vi "Oxford-1820-Main.vi"() -> ()   [LabVIEW 2016]
uses:
  <instrlib>/Mercury iXX/Public/Controls/Unit String.ctl
  <instrlib>/Mercury iXX/Public/Libraries/Heater/Controls/Heater Device (Read).ctl
  <instrlib>/Mercury iXX/Public/Controls/Manufacturing Data.ctl
  <instrlib>/Mercury iXX/Public/Libraries/Heater/Controls/Heater Signals Cluster.ctl
  <instrlib>/Mercury iXX/Public/Libraries/Level Meter/Controls/Level Meter (Read).ctl
  <instrlib>/Mercury iXX/Public/Libraries/Level Meter/Controls/Nitrogen Configuration.ctl
  <instrlib>/Mercury iXX/Public/Libraries/Level Meter/Controls/Frequency Configuration.ctl
  <instrlib>/Mercury iXX/Public/Libraries/Level Meter/Controls/Signals.ctl
  <instrlib>/Mercury iXX/Public/Libraries/Level Meter/Controls/Helium Configuration.ctl
  <instrlib>/Mercury iXX/Public/Libraries/Level Meter/Controls/Resistance Configuration.ctl
  <instrlib>/Mercury iXX/Public/Libraries/Level Meter/Controls/Pre-Pulse.ctl
  <instrlib>/Mercury iXX/Public/Libraries/Level Meter/Controls/Pulse.ctl
  <instrlib>/Mercury iXX/Public/Libraries/Auxiliary/Controls/AUX Device (Read).ctl
  <instrlib>/Mercury iXX/Public/Libraries/Auxiliary/Controls/AUX Signals (Read).ctl
  <instrlib>/Mercury iXX/Public/Libraries/Magnet/Controls/Device (Read).ctl
  <instrlib>/Mercury iXX/Public/Libraries/Magnet/Controls/Signals (Read).ctl
  <instrlib>/Mercury iXX/Public/Libraries/Magnet/Controls/Identifier.ctl
  <instrlib>/Mercury iXX/Public/Libraries/Temperature/Controls/Calibration Cluster.ctl
  <instrlib>/Mercury iXX/Public/Libraries/Temperature/Controls/Calibration Interpolation.ctl
  <instrlib>/Mercury iXX/Public/Libraries/Temperature/Controls/Excitation Cluster.ctl
  <instrlib>/Mercury iXX/Public/Libraries/Temperature/Controls/Excitation Type.ctl
  <instrlib>/Mercury iXX/Public/Libraries/Pressure/Controls/Pressure Signals Cluster.ctl
  <instrlib>/Mercury iXX/Public/Controls/Mercury Reference.ctl
  <instrlib>/Mercury iXX/Public/Controls/Comms Transport Layer.ctl
  <instrlib>/Mercury iXX/Private/Controls/Query Dynamic Reference.ctl
  <userlib>/LevyLab/Oxford 1820 API/Typedefs/Status.ctl
  <instrlib>/Mercury iXX/Public/Libraries/Magnet/Controls/PSU Actions.ctl
  <instrlib>/Mercury iXX/Public/Libraries/System/Controls/User Mode.ctl
  <instrlib>/Mercury iXX/Public/Libraries/Magnet/Controls/Switch Heater.ctl
  <instrlib>/Mercury iXX/Public/Controls/ISOBus Address.ctl
  <instrlib>/Mercury iXX/Public/Controls/Response String.ctl
  <userlib>/_OpenG.lib/error/error.llb/Filter Error Codes (Array)__ogtk.vi
  <instrlib>/Mercury iXX/Public/Libraries/System/Open/Open System.vi
  <instrlib>/Mercury iXX/Public/Libraries/System/Read/Catalogue (Read).vi
  <instrlib>/Mercury iXX/Public/Libraries/System/Read/Display Automatic Dimming (Read).vi
  <instrlib>/Mercury iXX/Public/Libraries/System/Read/Display Automatic Dimming Time (Read).vi
  <instrlib>/Mercury iXX/Public/Libraries/System/Read/Display Brightness (Read).vi
  <instrlib>/Mercury iXX/Public/Libraries/System/Read/Date (Read).vi
  <instrlib>/Mercury iXX/Public/Libraries/System/Read/Time (Read).vi
  <instrlib>/Mercury iXX/Public/Libraries/System/Read/DateTime (Read).vi
  <instrlib>/Mercury iXX/Public/Libraries/System/Read/HVer (Read).vi
  <instrlib>/Mercury iXX/Public/Libraries/System/Read/FVer (Read).vi
  <instrlib>/Mercury iXX/Public/Libraries/System/Read/Serial Number (Read).vi
  <instrlib>/Mercury iXX/Public/Libraries/System/Read/Flash Space (Read).vi
  <instrlib>/Mercury iXX/Public/Libraries/System/Read/Mode (Read).vi
  <instrlib>/Mercury iXX/Public/Libraries/System/Set/DateTime (Set).vi
  <instrlib>/Mercury iXX/Public/Libraries/Temperature/Open/Open Temperature Device.vi
  <instrlib>/Mercury iXX/Public/Libraries/Temperature/Configuration/Read/Serial Number (Read).vi
  <instrlib>/Mercury iXX/Public/Libraries/Temperature/Configuration/Read/Nickname (Read).vi
  <instrlib>/Mercury iXX/Public/Libraries/Temperature/Configuration/Read/Excitation Magnitude (Read).vi
  <instrlib>/Mercury iXX/Public/Libraries/Temperature/Configuration/Read/Temperature Sensor (Read).vi
  <instrlib>/Mercury iXX/Public/Libraries/Temperature/Configuration/Read/Excitation Type (Read).vi
  <instrlib>/Mercury iXX/Public/Libraries/Temperature/Configuration/Read/Calibration Hot Limit (Read).vi
  <instrlib>/Mercury iXX/Public/Libraries/Temperature/Configuration/Read/Calibration Cold Limit (Read).vi
  <instrlib>/Mercury iXX/Public/Libraries/Temperature/Signals/Read/Voltage (Read).vi
  <instrlib>/Mercury iXX/Public/Libraries/Temperature/Signals/Read/Temperature (Read).vi
  <instrlib>/Mercury iXX/Public/Libraries/Temperature/Configuration/Read/Temperature Device (Read).vi
  <instrlib>/Mercury iXX/Public/Libraries/Heater/Open/Open Heater Device.vi
  <instrlib>/Mercury iXX/Public/Libraries/Heater/Configuration/Read/Heater Device (Read).vi
  <instrlib>/Mercury iXX/Public/Libraries/Heater/Configuration/Read/Nickname (Read).vi
  <instrlib>/Mercury iXX/Public/Libraries/Heater/Configuration/Read/Serial Number (Read).vi
  <instrlib>/Mercury iXX/Public/Libraries/Heater/Configuration/Read/Voltage Limit (Read).vi
  <instrlib>/Mercury iXX/Public/Libraries/Heater/Configuration/Read/Nominal Resistance (Read).vi
  <instrlib>/Mercury iXX/Public/Libraries/Heater/Configuration/Read/Maximum Power (Read).vi
  <instrlib>/Mercury iXX/Public/Libraries/Heater/Signals/Read/Voltage (Read).vi
  <instrlib>/Mercury iXX/Public/Libraries/Heater/Signals/Read/Power (Read).vi
  <instrlib>/Mercury iXX/Public/Libraries/Heater/Signals/Read/Current (Read).vi
  <instrlib>/Mercury iXX/Public/Libraries/Auxiliary/Open/Open Auxiliary Device.vi
  <instrlib>/Mercury iXX/Public/Libraries/Auxiliary/Configuration/Read/Aux Device (Read).vi
  <instrlib>/Mercury iXX/Public/Libraries/Auxiliary/Configuration/Read/Serial Number (Read).vi
  <instrlib>/Mercury iXX/Public/Libraries/Auxiliary/Configuration/Read/Minimum Gas Flow (Read).vi
  <instrlib>/Mercury iXX/Public/Libraries/Auxiliary/Configuration/Read/Gas Flow Scaling (Read).vi
  <instrlib>/Mercury iXX/Public/Libraries/Auxiliary/Configuration/Read/Temperature Error Sensitivity (Read).vi
  <instrlib>/Mercury iXX/Public/Libraries/Auxiliary/Configuration/Read/Temperature Error Voltage Sensitivity (Read).vi
  <instrlib>/Mercury iXX/Public/Libraries/Auxiliary/Configuration/Read/Valve Gearing (Read).vi
  <instrlib>/Mercury iXX/Public/Libraries/Auxiliary/Configuration/Read/Stepper Speed (Read).vi
  <instrlib>/Mercury iXX/Public/Libraries/Auxiliary/Signals/Read/Position (Read).vi
  <instrlib>/Mercury iXX/Public/Libraries/Auxiliary/Signals/Read/Percent Open (Read).vi
  <instrlib>/Mercury iXX/Public/Libraries/Pressure/Open/Open Pressure Device.vi
  <instrlib>/Mercury iXX/Public/Libraries/Pressure/Configuration/Read/Pressure Device (Read).vi
  <instrlib>/Mercury iXX/Public/Libraries/Pressure/Configuration/Read/Nickname (Read).vi
  <instrlib>/Mercury iXX/Public/Libraries/Pressure/Signals/Read/Current (Read).vi
  <instrlib>/Mercury iXX/Public/Libraries/Pressure/Signals/Read/Voltage (Read).vi
  <instrlib>/Mercury iXX/Public/Libraries/Level Meter/Open/Open Level Meter Device.vi
  <instrlib>/Mercury iXX/Public/Libraries/Level Meter/Configuration/Read/Level Meter Device (Read).vi
  <instrlib>/Mercury iXX/Public/Libraries/Level Meter/Configuration/Read/Serial Number (Read).vi
  <instrlib>/Mercury iXX/Public/Libraries/Level Meter/Configuration/Read/Helium Probe Resistance (Read).vi
  <instrlib>/Mercury iXX/Public/Libraries/Level Meter/Configuration/Read/Helium Pulse Mag (Read).vi
  <instrlib>/Mercury iXX/Public/Libraries/Level Meter/Configuration/Read/Helium Pulse Duration (Read).vi
  <instrlib>/Mercury iXX/Public/Libraries/Level Meter/Configuration/Read/Nitrogen Freq at 100 (Read).vi
  <instrlib>/Mercury iXX/Public/Libraries/Level Meter/Configuration/Read/Nitrogen Pulse Count Period (Read).vi
  <instrlib>/Mercury iXX/Public/Libraries/Level Meter/Signals/Read/Probe Resistance Helium (Read).vi
  <instrlib>/Mercury iXX/Public/Libraries/Level Meter/Signals/Read/Probe Level Helium (Read).vi
  <instrlib>/Mercury iXX/Public/Libraries/Level Meter/Signals/Read/Probe Count Nitrogen (Read).vi
  <instrlib>/Mercury iXX/Public/Libraries/Level Meter/Signals/Read/Probe Level Nitrogen (Read).vi
  <instrlib>/Mercury iXX/Public/Libraries/Magnet/Open/Open Magnet Device.vi
  <instrlib>/Mercury iXX/Public/Libraries/Magnet/Configuration/Read/Magnet Device (Read).vi
  <instrlib>/Mercury iXX/Public/Libraries/Magnet/Configuration/Read/Serial Number (Read).vi
  <instrlib>/Mercury iXX/Public/Libraries/Magnet/Configuration/Read/Bipolar Output (Read).vi
  <instrlib>/Mercury iXX/Public/Libraries/Magnet/Configuration/Read/Output Configuration (Read).vi
  <instrlib>/Mercury iXX/Public/Libraries/Magnet/Configuration/Read/Current Limit (Read).vi
  <instrlib>/Mercury iXX/Public/Libraries/Magnet/Configuration/Read/Current to Field Factor (Read).vi
  <instrlib>/Mercury iXX/Public/Libraries/Magnet/Configuration/Read/Switch Present (Read).vi
  <instrlib>/Mercury iXX/Public/Libraries/Magnet/Configuration/Read/Software Voltage Limit (Read).vi
  <instrlib>/Mercury iXX/Public/Libraries/Magnet/Signals/Read/Current Rate (Read).vi
  <instrlib>/Mercury iXX/Public/Libraries/Magnet/Configuration/Read/PSU Action Status (Read).vi
  <instrlib>/Mercury iXX/Public/Libraries/Temperature/Signals/Read/Resistance (Read).vi
  <instrlib>/Mercury iXX/Public/Libraries/Temperature/Configuration/Set/Excitation Magnitude (Set).vi
  <instrlib>/Mercury iXX/Public/Libraries/Magnet/Signals/Read/Switch Heater Status (Read).vi
  <instrlib>/Mercury iXX/Public/Libraries/Magnet/Signals/Read/Current (Read).vi
  <instrlib>/Mercury iXX/Public/Libraries/Magnet/Signals/Read/Voltage (Read).vi
  <instrlib>/Mercury iXX/Public/Libraries/Magnet/Signals/Read/Field (Read).vi
  <instrlib>/Mercury iXX/Public/Libraries/Magnet/Signals/Read/Target Field Rate (Read).vi
  <instrlib>/Mercury iXX/Public/Libraries/Magnet/Signals/Read/Target Field (Read).vi
  <instrlib>/Mercury iXX/Public/Libraries/Magnet/Signals/Read/Persistant Field (Read).vi
  <instrlib>/Mercury iXX/Public/Libraries/Magnet/Configuration/Set/PSU Action Status (Set).vi
  <instrlib>/Mercury iXX/Public/Libraries/System/Set/Mode (Set).vi
  <instrlib>/Mercury iXX/Public/Libraries/Magnet/Configuration/Set/Switch Heater Current (Set).vi
  <instrlib>/Mercury iXX/Public/Libraries/Magnet/Signals/Read/Persistant Current (Read).vi
  <instrlib>/Mercury iXX/Public/Libraries/Magnet/Signals/Set/Switch Heater No Check (Set).vi
  <instrlib>/Mercury iXX/Public/Libraries/Magnet/Signals/Set/Target Field Rate (Set).vi
  <instrlib>/Mercury iXX/Public/Libraries/Magnet/Signals/Set/Target Field (Set).vi
  <instrlib>/Mercury iXX/Public/Libraries/Lambda/Open/Open Lambda Device.vi
  <instrlib>/Mercury iXX/Public/Libraries/Lambda/Configuration/Set/Lambda Flow Auto (Set).vi
  <instrlib>/Mercury iXX/Public/Libraries/Level Meter/Configuration/Set/Pulse Slow-Fast (Set).vi
  <instrlib>/Mercury iXX/Public/Libraries/Lambda/Configuration/Set/Lambda Percentage Flow (Set).vi
  <instrlib>/Mercury iXX/Mercury iXX.lvlib
  <instrlib>/Mercury iXX/Public/Libraries/Pressure.lvlib
  <instrlib>/Mercury iXX/Public/Libraries/System.lvlib
  <instrlib>/Mercury iXX/Public/Libraries/Temperature.lvlib
  <instrlib>/Mercury iXX/Public/Libraries/Auxiliary.lvlib
  <instrlib>/Mercury iXX/Public/Libraries/Magnet.lvlib
  <instrlib>/Mercury iXX/Public/Libraries/Level Meter.lvlib
  <instrlib>/Mercury iXX/Public/Libraries/Lambda.lvlib
  <userlib>/LevyLab/Oxford 1820 API/Mercury-1820-API.lvlib
  <instrlib>/Mercury iXX/Public/Libraries/Heater.lvlib
panel:
  in  "Tab Control":T1(tab)
  in  "Enable RS232 Panel":bool
  out "LEDs":bool[](array[boolean])
  out "Iteration Time":dbl
  in  "Percentage Open":dbl=100.0 format="%#_13g"
  out "PS Heat on or off (sec)":dbl format="%<%H:%M:%S>t"
  out "LPF on (sec)":dbl=5373.0 format="%<%H:%M:%S>t"
  out "Magnet Status 2":string
  in  "OK":bool
  out "LPF Resistance":dbl=4.2075 format="%_3f ohms"
  out "Magnet Resistance":dbl=3.8705 format="%_3f ohms"
  out "ETA":timestamp format="%<%I:%M:%S %p\n%m/%d/%y>T"
  in  "Open Needle Valve":bool
  in  "Close Needle Valve":bool
  in  "Lambda":bool
  out "LPF Pressure":dbl format="%_5f mB"
  out "LPF Needle Valve (%)":dbl format="%_6g"
  out "LPF Temperature":dbl=4.2075 format="%_2f K"
  out "Magnet Temperature":dbl=3.8705 format="%_2f K"
  out "He LVL Chart":dbl(slide)=52.0833 scale=0.0..100.0
  out "N2 LVL Chart":dbl(slide)=61.3025 scale=0.0..100.0
  in  "Remote Mode":bool
  out "Power Supply Field (T)":dbl=0.0001 format="%#.5f"
  out "Magnet Field (T)":dbl format="%.5f"
  out "Voltage (V)":dbl=-0.0003 format="%.5f"
  out "Current (A)":dbl=0.0006 format="%.5f"
  out "N2 LEVEL":dbl=61.3025 format="%.0f %"
  out "He LEVEL":dbl=52.0833 format="%.0f %"
  in  "Fast/Slow Fill":bool
  out "Magnet Field (T)":dbl(knob) caption="Voltage (V)" scale=-20.0..20.0
  out "SWITCH HEATER":bool
  in  "PS Heat":bool
  in  "Clamp":bool
  in  "To Set":bool
  in  "To Zero":bool
  in  "Hold":bool
  out "Magnet Status":string="Clamped"
  out "Target Field Rate (T/min)":dbl=1.0 format="%.5f"
  out "Target Field (T)":dbl format="%#.5f"
  in  "Target Rate (T/min)":dbl=0.1 format="%.5f"
  in  "Target Field (T)":dbl format="%#.5f"
  in  "Send to IPS":bool
  out "Voltage (V)":dbl(knob)=-0.0003 scale=-10.0..10.0
  out "Current (A)":dbl(knob)=0.0006 scale=-180.0..180.0
  in  "Mercury Functions":T2(tab)=enum."ITC: Temperature"
  out "time stamp":timestamp=timestamp(3543841780 s since 1904-01-01)
  out "Free Space":i32=166384 caption="Free Space (KB)"
  out "Set Date Response":string="VALID"
  out "String":string="NORM" caption="User Mode"
  out "Date":string="2016:04:18"
  out "Time":string="11:29:40"
  out "Hardware Version":string="65"
  out "Firmware Version":string="2.2.6.20"
  out "Serial Number":string="154650110"
  out "ITC Devices":string[](array[string])=["DB4.G1:AUX", "DB8.P1:PRES", "MB0.H1:HTR", "MB1.T1:TEMP"]
  out "S/W Version(s)":string[](array[string])=["2.2.6.20\n"]
  out "Serial Number(s)":string[](array[string])=["154650110"]
  out "# of Instruments":i32=1
  out "Automatic Dimming":string="OFF"
  out "Dimming Time":string="5"
  out "Display Brightness":string="100"
  in  "ITC IP Address":string="130.49.180.101"
  out "Excitation Magnitude":dbl=5.0
  out "Sensor Type":string="NTC"
  out "Excitation Type":string="UNIP"
  out "Hot Limit":dbl=1000.0
  out "H Unit":T3="K"
  out "Cold Limit":dbl=1000.0
  out "C Unit":T3="K"
  out "Unit":T3
  out "Voltage":dbl=0.005
  out "V Unit":T3="V"
  out "Temperature":dbl=4.2075
  out "T Unit":T3="K"
  out "Temp S/N":string="154650110"
  out "T Nickname":string="Mag_AB_MB1"
  out "ITC Calibration":T4
  out "ITC Excitation":T6
  out "ITC Manufacturing":T8
  out "Heater Device Settings":T9={"Manufacturing"={"Hardware Version"="65", "Firmware Version"="2.3", "Serial Number"="154650110"}, "Nickname"="MB0.H1", "Voltage Limit"="1", "Nominal Resistance"="10", "Maximum Power"="0.1000", "Heater Signals"={"Voltage"="0.0507V", "Current"="-0.0000A", "Power"="0.0000W"}, "Status"="2"}
  out "Htr C Unit":T3="A"
  out "Htr P Unit":T3="W"
  out "Htr V Unit":T3="V"
  out "Htr Current":dbl=-0.0
  out "Htr Power":dbl
  out "Htr Voltage":dbl=0.0507
  out "Power Unit":T3
  out "Volt Unit":T3
  out "Res Unit":T3
  out "Maximum Power":dbl=0.1
  out "Htr Resistance":dbl=10.0
  out "Htr Voltage Limit":dbl=1.0
  out "Htr S/N":string="154650110"
  out "Htr Nickname":string="MB0.H1"
  out "Nickname":string="Lam_P_DB8"
  out "Current":dbl=-0.0
  out "Voltage":dbl=-8.219999999999999e-05
  out "Manufacturing":T8
  out "Pressure Signals":T11
  out "Auxiliary Device Details":T12={"Manufacturing"={"Hardware Version"="65", "Firmware Version"="3.1", "Serial Number"="154650084"}, "Min Flow"=0.0, "Scaling Factor"=50.0, "Temp Err"=9.0, "Temp V Err"=11.0, "Gear"=2, "Speed"=2, "Signals"={"Position"=0.0, "% Open"=0.0, "I0"="ON", "I1"="OFF", "I2"="OFF", "I3"="OFF", "O0"="OFF", "O1"="OFF", "O2"="OFF", "O3"="OFF"}, "Nickname"="DB4.G1", "Status"="0"} {"Signals"."% Open" min=0.0 max=100.0 step=0.1 format="%.4f"; "Signals"."Position" max=20.0 step=1.0 format="%.4f"; "Speed" max=7 step=1; "Gear" max=7 step=1; "Temp V Err" min=0.0 max=20.0 step=0.1; "Temp Err" min=0.0 max=20.0 step=0.1; "Scaling Factor" min=0.0 max=99.0 step=0.1; "Min Flow" min=0.0 max=20.0 step=0.1}
  out "Aux S/N":string="154650084"
  out "Min Flow":dbl caption="Minimum Gas Flow" format="%#.1f"
  out "Scaling Factor":dbl=50.0 caption="Gas Flow Scaling Factor" format="%#.1f"
  out "Temp Err":dbl=9.0 caption="Temperature Error Sensitivity" format="%#.1f"
  out "Temp V Err":dbl=11.0 caption="Temperature Voltage Error Sensitivity" format="%#.1f"
  out "Gear":u32=2 caption="Valve Gearing"
  out "Speed":u32=2 caption="Stepper Speed"
  out "Unit 2":T3
  out "Unit 3":T3
  out "Unit 4":T3
  out "Unit 5":T3
  out "Unit 6":T3
  out "Unit 7":T3
  out "Position":u32
  out "% Open":dbl caption="Percentage Open (%)"
  out "Unit":T3
  out "Unit":T3="%"
  out "time stamp 2":timestamp=timestamp(3543841781 s since 1904-01-01)
  out "Free Space 2":i32=166316 caption="Free Space (KB)"
  out "Set Date Response 2":string="VALID"
  out "String 2":string="NORM" caption="User Mode"
  out "Date 2":string="2016:04:18"
  out "Time 2":string="11:29:45"
  out "Hardware Version 2":string="65"
  out "Firmware Version 2":string="2.2.6.20"
  out "Serial Number 2":string="153350063"
  out "IPS Devices":string[](array[string])=["DB3.L1:LVL", "GRPX:PSU", "GRPY:PSU", "GRPZ:PSU", "MB1.T1:TEMP", "PSU.M1:PSU", "PSU.M2:PSU", "PSU.M3:PSU"]
  out "S/W Version(s) 2":string[](array[string])=["2.2.6.20\n"]
  out "Serial Number(s) 2":string[](array[string])=["153350063"]
  out "# of Instruments 2":i32=1
  out "Automatic Dimming 2":string="OFF"
  out "Dimming Time 2":string="5"
  out "Display Brightness 2":string="100"
  in  "IPS IP Address":string="130.49.180.102"
  out "LVL Device DetailSettings":T14={"Manufacturing"={"Hardware Version"="65", "Firmware Version"="2.2", "Serial Number"="152450013"}, "Nitrogen Configuration"={"Frequency Configuration"={"Freq 0%"=0.0, "Freq 100%"=0.0}, "Pulse Period"=0.0}, "Signals"={"Helium Signals"={"Resistance"=75.5626, "Level"=52.0833}, "Nitrogen Signals"={"Count"=8800.0, "Freq"=487361.0, "Level"=61.3445}}, "Nickname"="DB3.L1", "Status"="0", "Helium Configuration"={"Resistance Configuration"={"Res 0%"=0.0, "Res 100%"=0.0}, "Pre-Pulse"={"Magnitude"=0.0, "Duration"=0.0}, "Pulse"={"Magnitude"=0.0, "Duration"=0.0, "Delay"=0.0}}}
  out "LVL S/N":string="152450013"
  out "LVL P Magnitude":dbl=125.0 caption="Pulse Magnitude (mA)"
  out "LVL P Duration":dbl=5.0 caption="Pulse Duration (s)"
  out "N Freq 100%":dbl=7880.0 caption="Frequency at 100% (Hz)"
  out "N Pulse Period":dbl=1000.0 caption="Pulse Period (ms)"
  out "He Res Config":T19={"Res 0%"=149.0, "Res 100%"=8.0}
  out "He Resistance":dbl=75.5626 caption="Resistance (Ohms)"
  out "He Level":dbl=52.0833 caption="Helium Level (%)"
  out "N Counter":u32 caption="Counter"
  out "N Level":dbl=61.3445 caption="Nitrogen Level (%)"
  out "Excitation Magnitude 2":dbl=5.0
  out "Sensor Type 2":string="NTC"
  out "Excitation Type 2":string="UNIP"
  out "Hot Limit 2":dbl=1000.0
  out "H Unit 2":T3="K"
  out "Cold Limit 2":dbl=1000.0
  out "C Unit 2":T3="K"
  out "Unit 12":T3
  out "Voltage 2":dbl=0.005
  out "V Unit 2":T3="V"
  out "Temperature 2":dbl=3.8706
  out "T Unit 2":T3="K"
  out "Temp S/N 2":string="153350063"
  out "T Nickname 2":string="MB1.T1"
  out "IPS Calibration":T4
  out "IPS Excitation":T6
  out "IPS Manufacturing":T8
  out "Magnet Device Details":T22={"Manufacturing"={"Hardware Version"="NOT_FOUND", "Firmware Version"="NOT_FOUND", "Serial Number"="NOT_FOUND"}, "Nickname"="GRPZ", "Bipolar Output"="ON", "String"="PARA", "Current Limit"=174.0, "AtoB"=8.688, "Inductance"=39.406, "Switch Present"="PSU.M1", "Swh Htr Current"=86.0, "SW VLIM"=9.0, "V Trans Time"=1000.0, "Magnet PSU Signals"={"Voltage"=-0.0002, "Current"=0.0002, "Current Rate"=100.0, "Field"=0.0001, "Field Rate"=11.5101, "Persistant Current"=0.0003, "Persistant Field"=0.0, "Target Current"=0.0, "Target Field"=0.0, "Target Current Rate"=8.688, "Target Field Rate"=1.0, "Switch Heater Status (SWHT)"="OFF", "Switch Heater Status (SWHN)"="OFF"}, "PSU Action"="CLMP", "Status"="40000000", "Level Limit"=0.0, "Temperature Limit"=999.0} {"Temperature Limit" format="%#.1f"; "Level Limit" format="%#.1f"; "V Trans Time" format="%#.1f"; "SW VLIM" format="%#.1f"; "Swh Htr Current" format="%#.1f"; "Inductance" format="%#.1f"; "AtoB" format="%#.1f"; "Current Limit" format="%#.1f"}
  out "Mag S/N":string="NOT_FOUND"
  out "Bipolar Output":string="ON"
  out "Out Config":string="PARA" caption="Output Configuration"
  out "Current Limit":dbl=174.0 caption="Current Limit (A)" format="%#.1f"
  out "AtoB":dbl=8.688 caption="Current Field Factor (A/T)" format="%#.1f"
  out "Switch Present":string="PSU.M1"
  out "SW VLIM":dbl=9.0 caption="Software Voltage Limit (V)" format="%#.1f"
  out "Unit 8":T3
  out "Unit 9":T3
  out "Unit 10":T3
  out "Current Rate":dbl=100.0
  out "PSU Act Stat":string="CLMP" caption="PSU Action Status"
  out "Unit 11":T3="A/min"
  in  "Device Identifier":T24="GRPZ"
  out "M3 Voltage":dbl
  out "M3 Current":dbl
  out "M2 Voltage":dbl
  out "M2 Current":dbl
  out "M1 Voltage":dbl
  out "M1 Current":dbl
  out "Error List":T25(array[cluster])
  out "PS ON/OFF":timestamp format="%<%I:%M:%S %p>T"
  in  "Heater Current":bool
  in  "Swh Htr Current (mA)":dbl=90.0 format="%#_13g"
  in  "LPF ON":timestamp
  # "v2018/06/11"
  # "Voltage (V)"
  # "Magnet (T)"
  # "Current (A)"
  # "Slow Rates\nCurrent Range (A)     Field Range (T)    Rate (T/min)\n0       -- 100        0    -- 11.5       0.91\n100     -- 150        11.5 -- 17.2       0.23\n150     -- 155.467    17.2 -- 18         0.11\n155.567 -- 172.471    18   -- 20         0.11"
  # "Fast Rates\nCurrent Range (A)     Field Range (T)    Rate (T/min)\n0       -- 155.467    0    -- 18         1.0\n155.567 -- 172.471    18   -- 20         0.25"
  # "ITC: 101\nIPS: 102\nIPS VR: 67"
  # "ITC: 101\nIPS: 102\nIPS VR: 67"
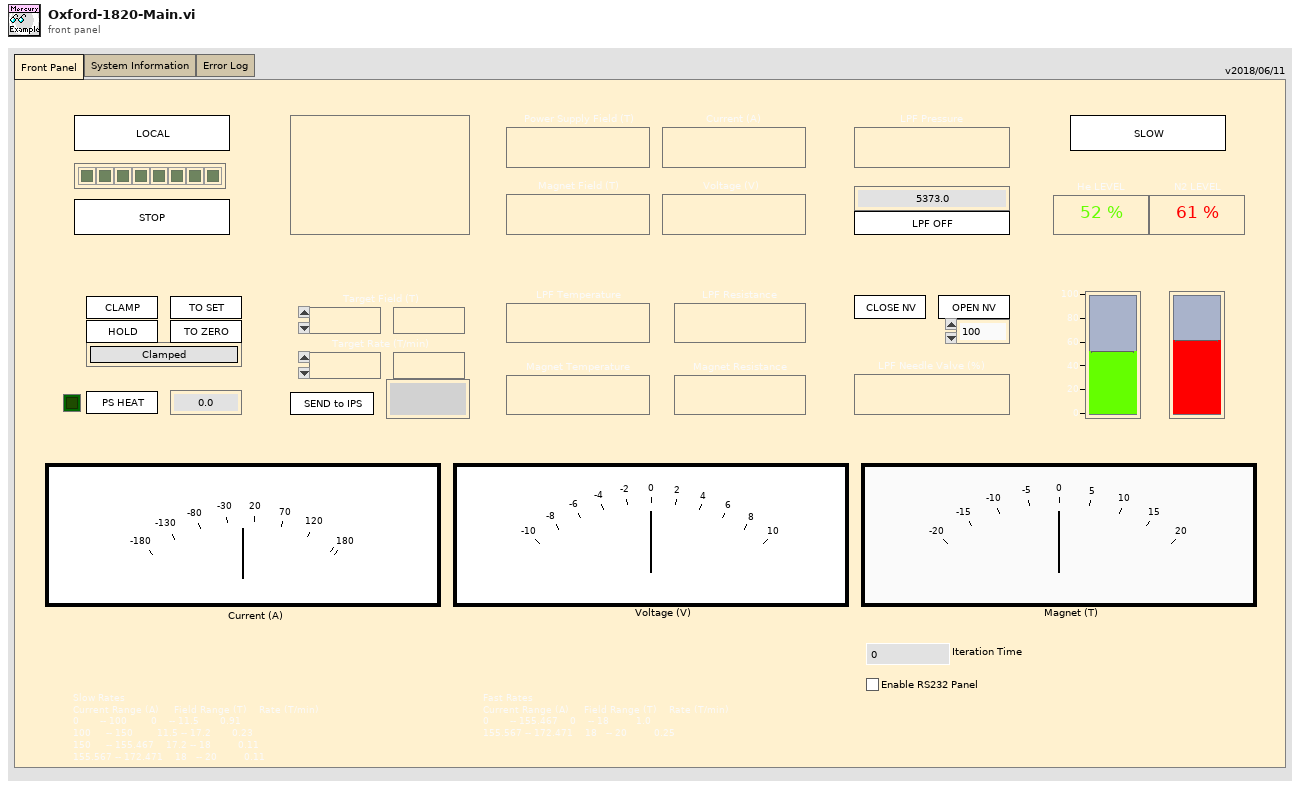
[diagram p1: front panel]
types:
  T1 = enum32{"Front Panel", "System Information", "Error Log"}
  T2 = enum32{"ITC: System", "ITC: Temperature", "ITC: Heater", "ITC: Pressure", "ITC: Auxiliary", "IPS: System", "IPS: Level Meter", "IPS: Temperature", "IPS: Magnet"}
  T3 = typedef "Mercury iXX.lvlib/Unit String.ctl" = string
  T4 = typedef "Mercury iXX.lvlib/Temperature.lvlib/Calibration Cluster.ctl" = cluster{"Filename":string, "Interpolation":T5, "Scaling Factor":string, "Offset Factor":string, "Hot Limit":string, "Cold Limit":string, "Last Calibration":string, "Reference":string}
  T5 = typedef "Mercury iXX.lvlib/Temperature.lvlib/Calibration Interpolation.ctl" = string
  T6 = typedef "Mercury iXX.lvlib/Temperature.lvlib/Excitation Cluster.ctl" = cluster{"Excitation Type":T7, "Magnitude":string}
  T7 = typedef "Mercury iXX.lvlib/Temperature.lvlib/Excitation Type.ctl" = string
  T8 = typedef "Mercury iXX.lvlib/Manufacturing Data.ctl" = cluster{"Hardware Version":string, "Firmware Version":string, "Serial Number":string}
  T9 = typedef "Mercury iXX.lvlib/Heater.lvlib/Heater Device (Read).ctl" = cluster{"Manufacturing":T8, "Nickname":string, "Voltage Limit":string, "Nominal Resistance":string, "Maximum Power":string, "Heater Signals":T10, "Status":string}
  T10 = typedef "Mercury iXX.lvlib/Heater.lvlib/Heater Signals Cluster.ctl" = cluster{"Voltage":string, "Current":string, "Power":string}
  T11 = typedef "Mercury iXX.lvlib/Pressure.lvlib/Pressure Signals Cluster.ctl" = cluster{"Voltage":string, "Current":string, "Power":string, "Pressure":string}
  T12 = typedef "Mercury iXX.lvlib/Auxiliary.lvlib/AUX Device (Read).ctl" = cluster{"Manufacturing":T8, "Min Flow":dbl, "Scaling Factor":dbl, "Temp Err":dbl, "Temp V Err":dbl, "Gear":u32, "Speed":u32, "Signals":T13, "Nickname":string, "Status":string}
  T13 = typedef "Mercury iXX.lvlib/Auxiliary.lvlib/AUX Signals (Read).ctl" = cluster{"Position":dbl, "% Open":dbl, "I0":string, "I1":string, "I2":string, "I3":string, "O0":string, "O1":string, "O2":string, "O3":string}
  T14 = typedef "Mercury iXX.lvlib/Level Meter.lvlib/Level Meter (Read).ctl" = cluster{"Manufacturing":T8, "Nitrogen Configuration":T15, "Signals":T17, "Nickname":string, "Status":string, "Helium Configuration":T18}
  T15 = typedef "Mercury iXX.lvlib/Level Meter.lvlib/Nitrogen Configuration.ctl" = cluster{"Frequency Configuration":T16, "Pulse Period":dbl}
  T16 = typedef "Mercury iXX.lvlib/Level Meter.lvlib/Frequency Configuration.ctl" = cluster{"Freq 0%":dbl, "Freq 100%":dbl}
  T17 = typedef "Mercury iXX.lvlib/Level Meter.lvlib/Signals.ctl" = cluster{"Helium Signals":cluster{"Resistance":dbl, "Level":dbl}, "Nitrogen Signals":cluster{"Count":dbl, "Freq":dbl, "Level":dbl}}
  T18 = typedef "Mercury iXX.lvlib/Level Meter.lvlib/Helium Configuration.ctl" = cluster{"Resistance Configuration":T19, "Pre-Pulse":T20, "Pulse":T21}
  T19 = typedef "Mercury iXX.lvlib/Level Meter.lvlib/Resistance Configuration.ctl" = cluster{"Res 0%":dbl, "Res 100%":dbl}
  T20 = typedef "Mercury iXX.lvlib/Level Meter.lvlib/Pre-Pulse.ctl" = cluster{"Magnitude":dbl, "Duration":dbl}
  T21 = typedef "Mercury iXX.lvlib/Level Meter.lvlib/Pulse.ctl" = cluster{"Magnitude":dbl, "Duration":dbl, "Delay":dbl}
  T22 = typedef "Mercury iXX.lvlib/Magnet.lvlib/Device (Read).ctl" = cluster{"Manufacturing":T8, "Nickname":string, "Bipolar Output":string, "String":string, "Current Limit":dbl, "AtoB":dbl, "Inductance":dbl, "Switch Present":string, "Swh Htr Current":dbl, "SW VLIM":dbl, "V Trans Time":dbl, "Magnet PSU Signals":T23, "PSU Action":string, "Status":string, "Level Limit":dbl, "Temperature Limit":dbl}
  T23 = typedef "Mercury iXX.lvlib/Magnet.lvlib/Signals (Read).ctl" = cluster{"Voltage":dbl, "Current":dbl, "Current Rate":dbl, "Field":dbl, "Field Rate":dbl, "Persistant Current":dbl, "Persistant Field":dbl, "Target Current":dbl, "Target Field":dbl, "Target Current Rate":dbl, "Target Field Rate":dbl, "Switch Heater Status (SWHT)":string, "Switch Heater Status (SWHN)":string}
  T24 = typedef "Mercury iXX.lvlib/Magnet.lvlib/Identifier.ctl" = string
  T25 = cluster{"time":timestamp, "code":i32, "source":string}[]
  T26 = enum32{"invalid app kind", "Development System", "Run Time System", "Student Edition", "Embedded LabVIEW", "Evaluation", "Custom"}
  T27 = cluster{"time":timestamp, "code":i32, "source":string}
  T28 = enum32{"Invalid", "Standard", "Closed", "Hidden", "Minimized", "Maximized"}
  T29 = typedef "Mercury-1820-API.lvlib/Status.ctl" = cluster{"Magnet Field":dbl, "PS Field":dbl, "Target Field":dbl, "Target Field Rate":dbl, "Voltage":dbl, "Current":dbl, "Switch":bool, "Mercury State":string}
  T30 = cluster{"Magnet Field":dbl, "PS Field":dbl, "Target Field":dbl, "Target Field Rate":dbl, "Voltage":dbl, "Current":dbl}
  T31 = typedef "Mercury iXX.lvlib/Magnet.lvlib/PSU Actions.ctl" = string
  T32 = typedef "Mercury iXX.lvlib/System.lvlib/User Mode.ctl" = string
  T33 = typedef "Mercury iXX.lvlib/Magnet.lvlib/Switch Heater.ctl" = string
  T34 = typedef "Mercury iXX.lvlib/ISOBus Address.ctl" = i32
  T35 = typedef "Mercury iXX.lvlib/Response String.ctl" = string
  T36 = typedef "Mercury iXX.lvlib/Mercury Reference.ctl" = cluster{"Comms":refnum<visa-resource-name>, "Device ID":string[], "Comms Layer":T37, "Command":string, "Query reference":T38}
  T37 = typedef "Mercury iXX.lvlib/Comms Transport Layer.ctl" = enum16{"Ethernet TCP/IP", "USB", "ISOBus - RS-232", "GPIB"}
  T38 = typedef "Mercury iXX.lvlib/Query Dynamic Reference.ctl" = refnum<vi>
  T39 = cluster{"Core":cluster{"Current VI Reference":refnum<vi>, "Close Panel on Exit?":bool}, "Mercury ITC Ref":T36, "Mercury IPS Ref":T36, "sentinel":bool, "Error Log":cluster{"time":timestamp, "code":i32, "source":string}[], "read ITC T?":bool, "counter":i32, "LEDs":bool[]}
  T40 = typedef "Filtered Error Details - Cluster__ogtk.ctl" = cluster{"code":i32, "source":string}
  T41 = cluster{"Current VI Reference":refnum<vi>, "Close Panel on Exit?":bool}
  T42 = typedef "Mercury iXX.lvlib/Temperature.lvlib/Temperature Sensor Type.ctl" = string
  T43 = typedef "Mercury iXX.lvlib/Temperature.lvlib/Temperature Device (Read).ctl" = cluster{"Manufacturing":T8, "Temperature Sensor Type":T42, "Excitation":T6, "Calibration":T4, "Control Loop":T44, "Temperature Signals":T45, "Nickname":string, "Status":string}
  T44 = typedef "Mercury iXX.lvlib/Temperature.lvlib/Loop Cluster.ctl" = cluster{"Heater":string, "Auxiliary":string, "Heater Auto":string, "Percentage Heat":string, "Temperature Set Point":string, "PID Auto (from file)":string, "P Value":string, "I Value":string, "D Value":string, "Auto PID Table Filename":string, "Flow Auto":string, "Target Heater Table":string, "Sweep mode":string, "Sweep Table Filename":string, "Percentage Flow":string}
  T45 = typedef "Mercury iXX.lvlib/Temperature.lvlib/Temperature Signals Cluster.ctl" = cluster{"Voltage":string, "Current":string, "Power":string, "Resistance":string, "Temperature":string, "Sensitivity":string, "Reference":string}
  T46 = typedef "Mercury iXX.lvlib/Pressure.lvlib/Pressure Device (Read).ctl" = cluster{"Manufacturing":T8, "Temperature Sensor Type":T47, "Calibration":T48, "Control Loop":T50, "Pressure Signals":T11, "Nickname":string, "Status":string}
  T47 = typedef "Mercury iXX.lvlib/Pressure.lvlib/Pressure Sensor Type.ctl" = string
  T48 = typedef "Mercury iXX.lvlib/Pressure.lvlib/Calibration Cluster.ctl" = cluster{"Filename":string, "Interpolation":T49, "Scaling Factor":string, "Offset Factor":string, "High Limit":string, "Low Limit":string, "Last Calibration":string}
  T49 = typedef "Mercury iXX.lvlib/Pressure.lvlib/Calibration Interpolation.ctl" = string
  T50 = typedef "Mercury iXX.lvlib/Pressure.lvlib/Loop Cluster.ctl" = cluster{"Heater":string, "Auxiliary":string, "Heater Auto":string, "Percentage Heat":string, "Pressure Set Point":string, "PID Auto (from file)":string, "P Value":string, "I Value":string, "D Value":string, "Auto PID Table Filename":string, "Flow Auto":string, "Target Heater Table":string, "Sweep mode":string, "Sweep Table Filename":string, "Percentage Flow":string}
  T51 = typedef "Mercury iXX.lvlib/Magnet.lvlib/Output Configuration.ctl" = string
  T52 = typedef "Mercury-1820-API.lvlib/Actions.ctl" = cluster{"Hold":bool, "Clamp":bool, "To Set":bool, "To Zero":bool, "Send to IPS":bool, "PS Heat":bool, "Lambda":bool}
  T53 = typedef "Mercury-1820-API.lvlib/Targets.ctl" = cluster{"Target Field (T)":dbl, "Target Field Rate (T/min)":dbl}
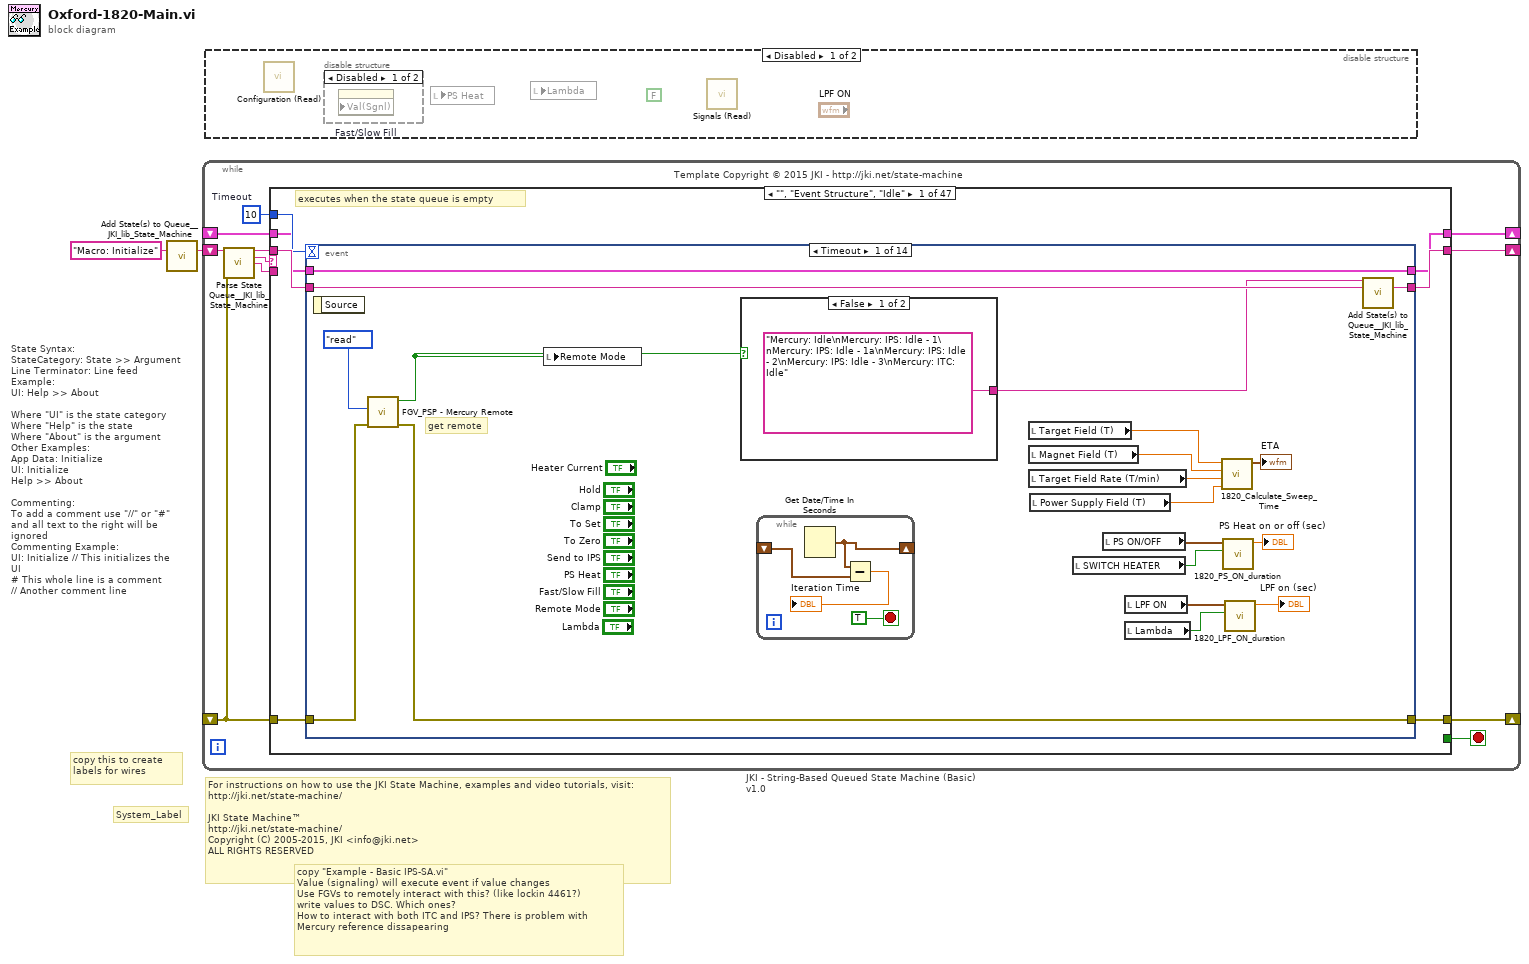
[diagram p0: block diagram]
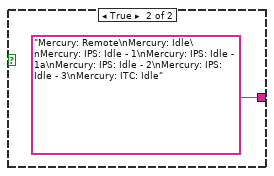
[diagram p4: hidden frame]
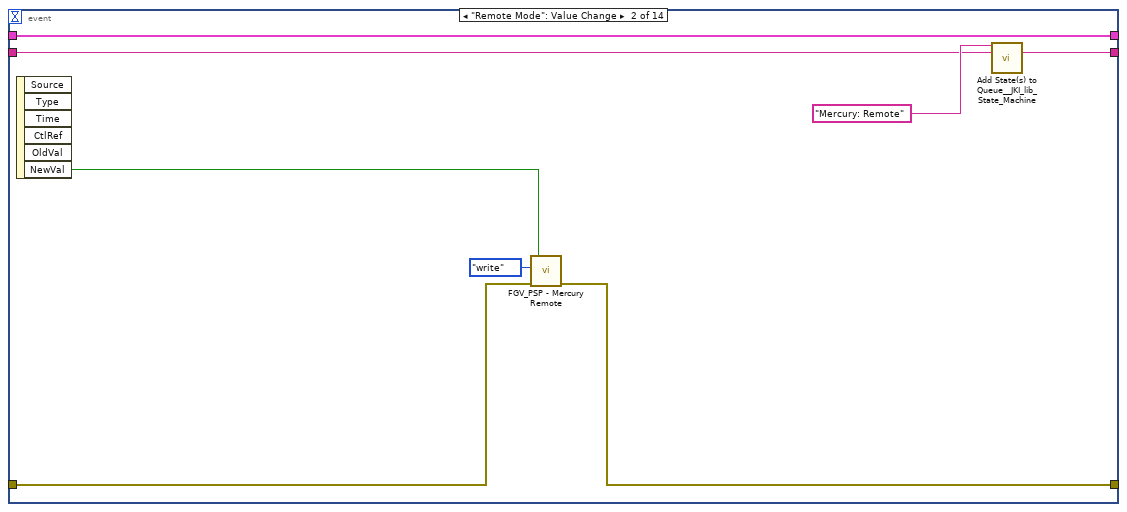
[diagram p5: hidden frame]
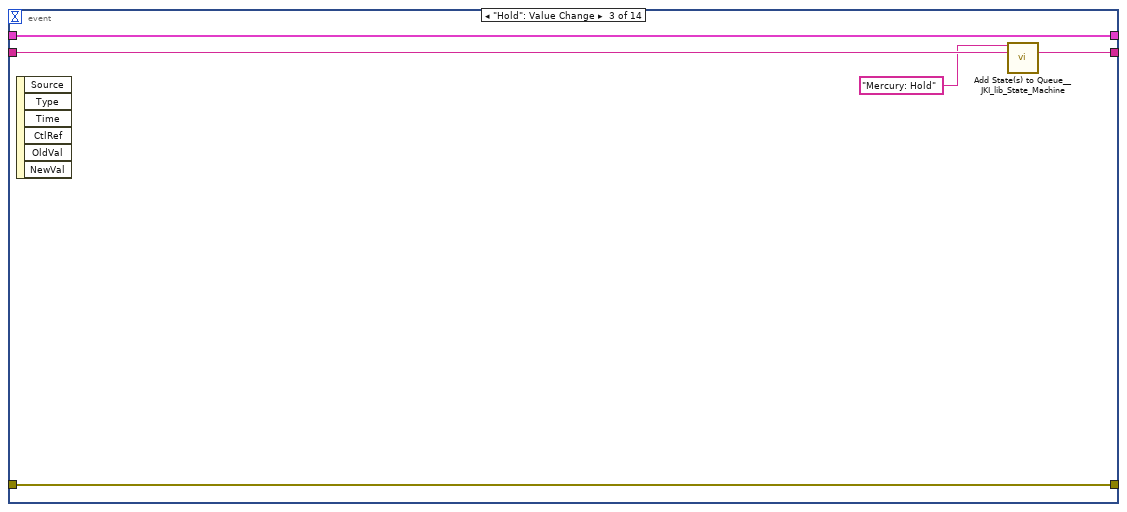
[diagram p6: hidden frame]
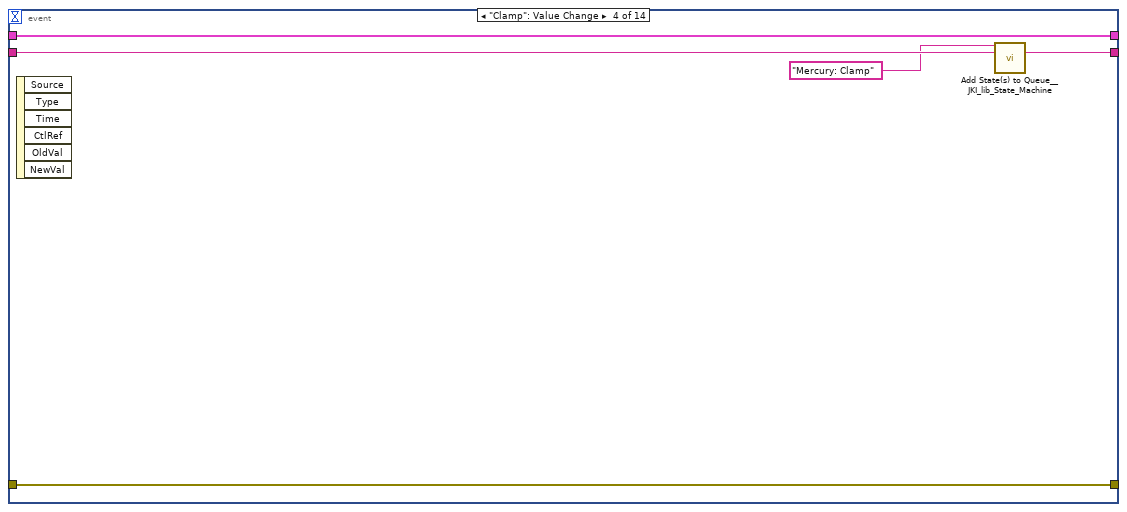
[diagram p7: hidden frame]
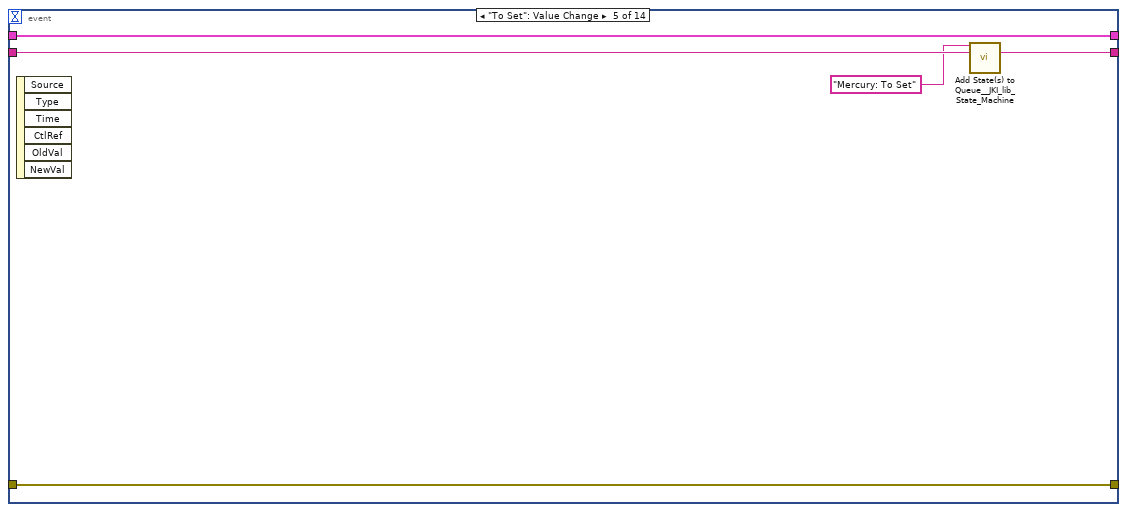
[diagram p8: hidden frame]
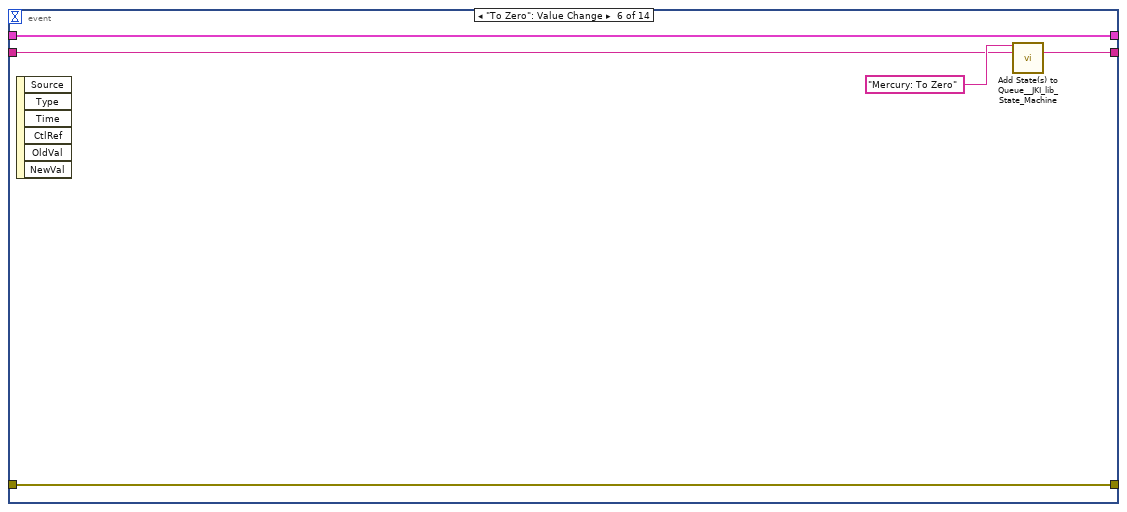
[diagram p9: hidden frame]
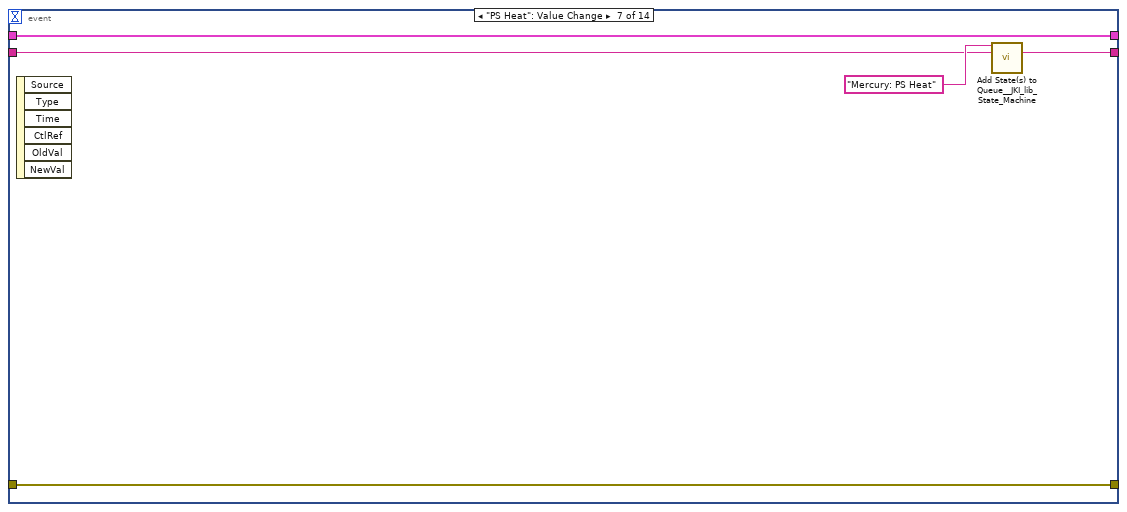
[diagram p10: hidden frame]
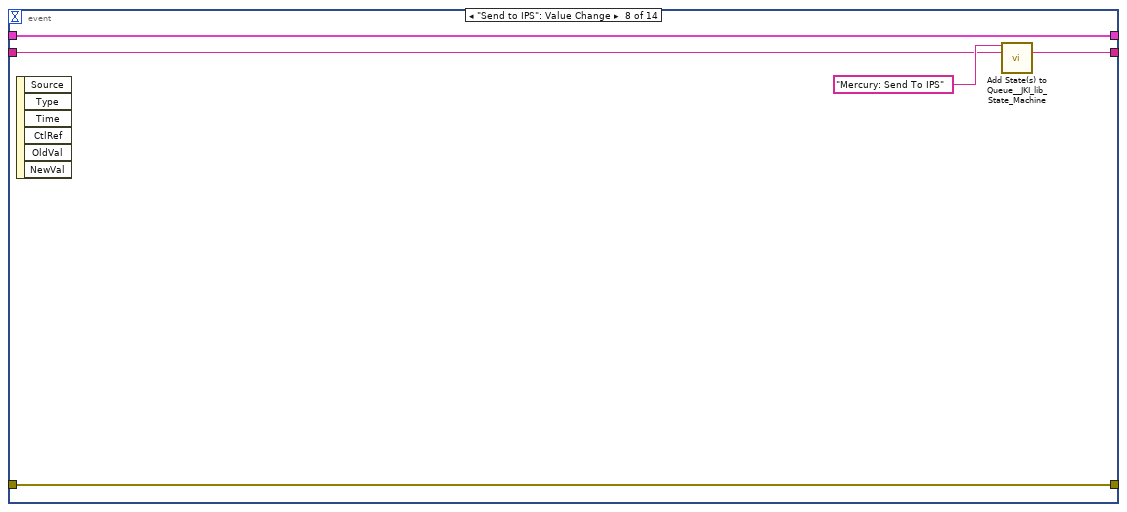
[diagram p11: hidden frame]
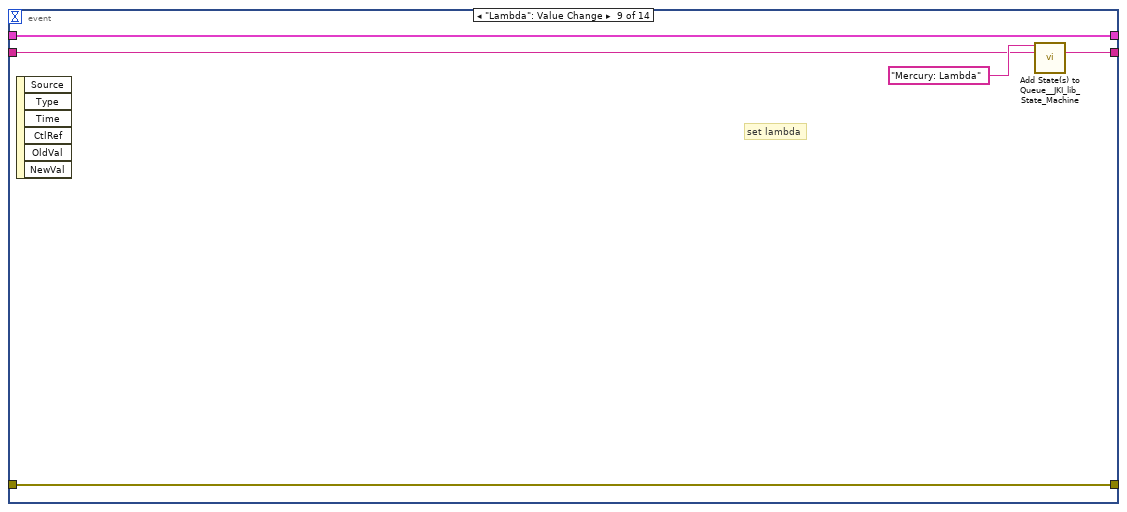
[diagram p12: hidden frame]
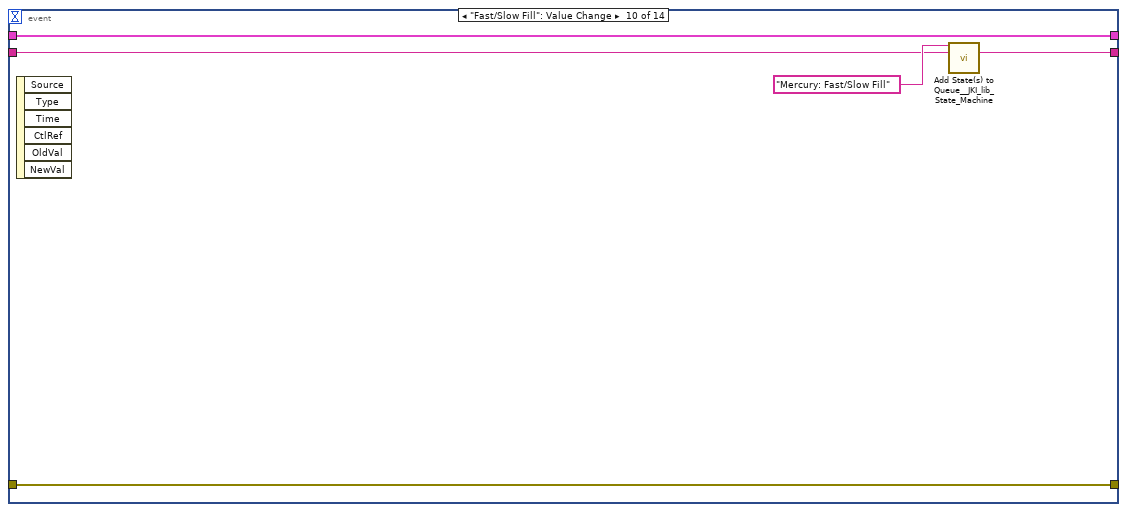
[diagram p13: hidden frame]
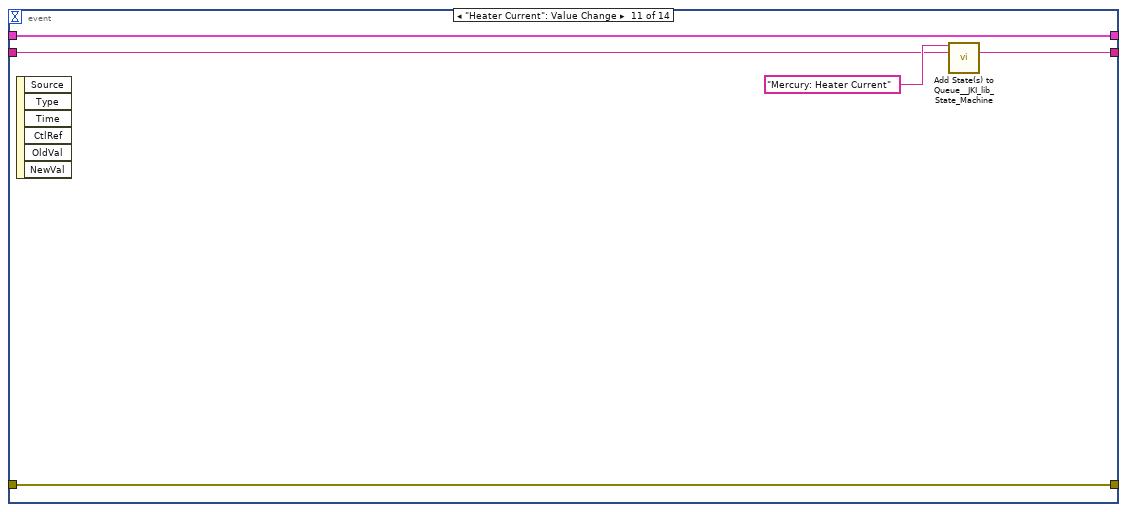
[diagram p14: hidden frame]
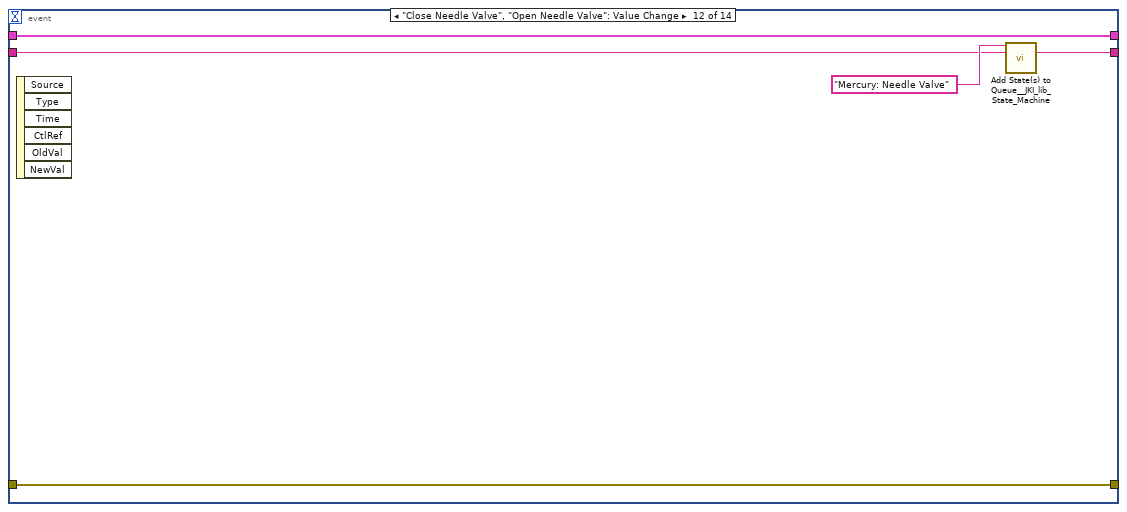
[diagram p15: hidden frame]
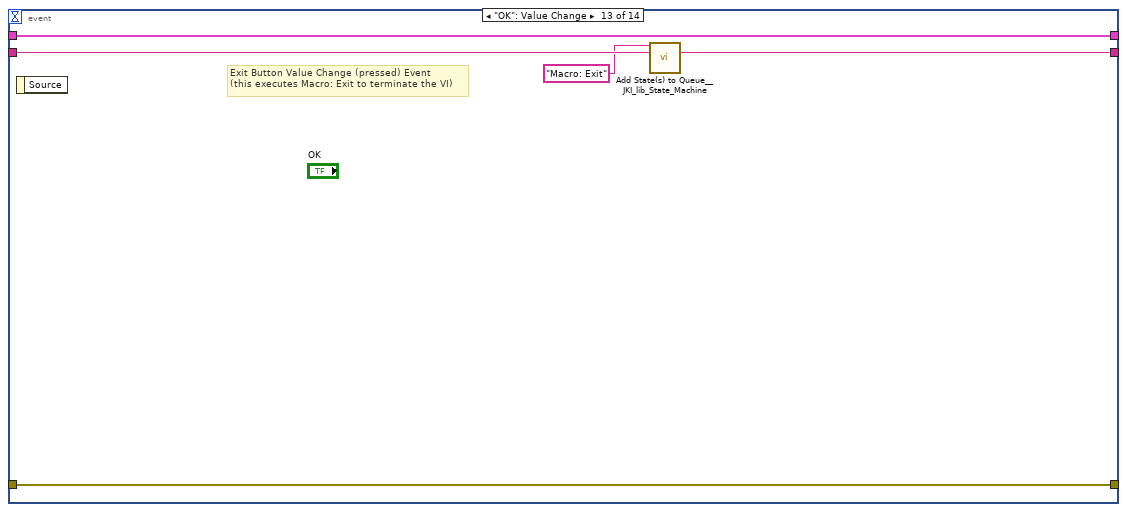
[diagram p16: hidden frame]
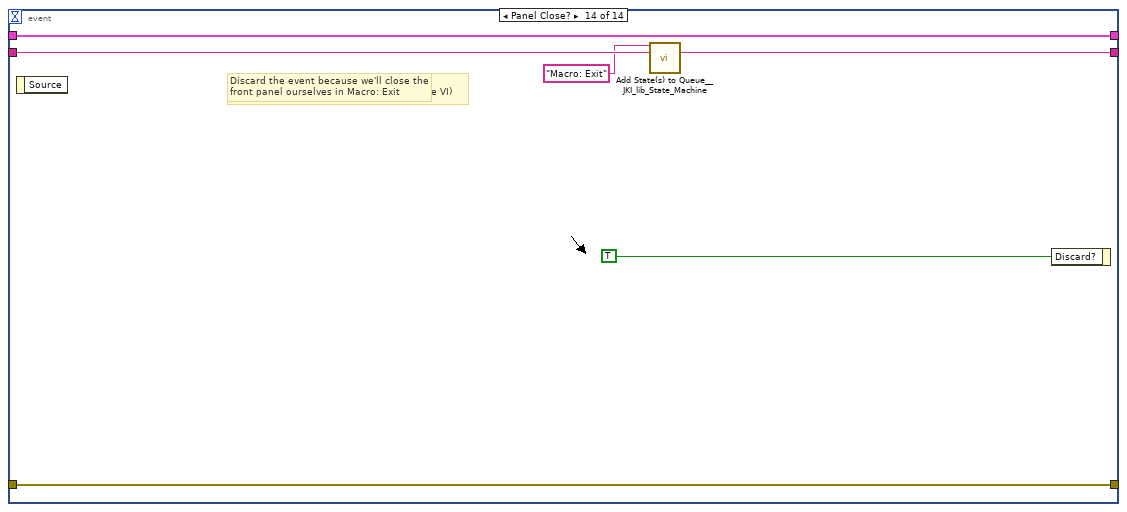
[diagram p17: hidden frame]
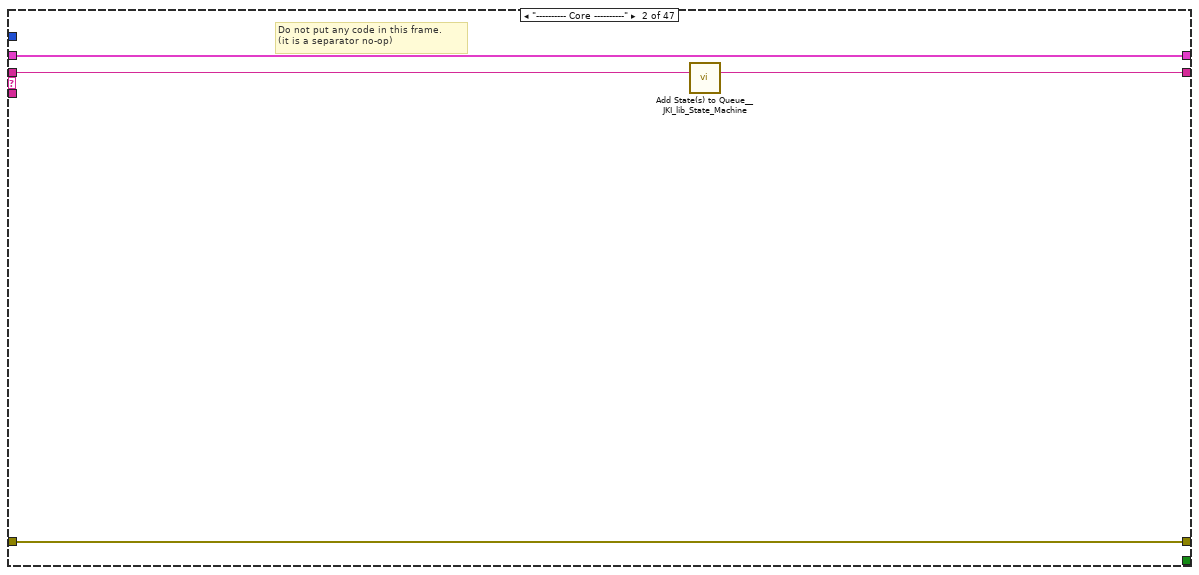
[diagram p18: hidden frame]
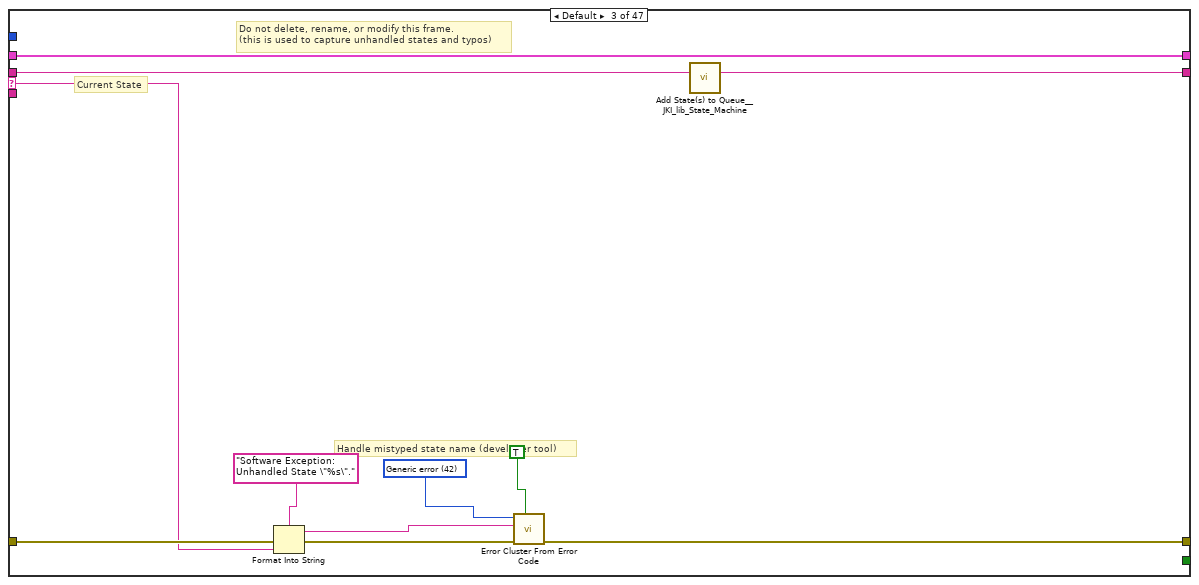
[diagram p19: hidden frame]
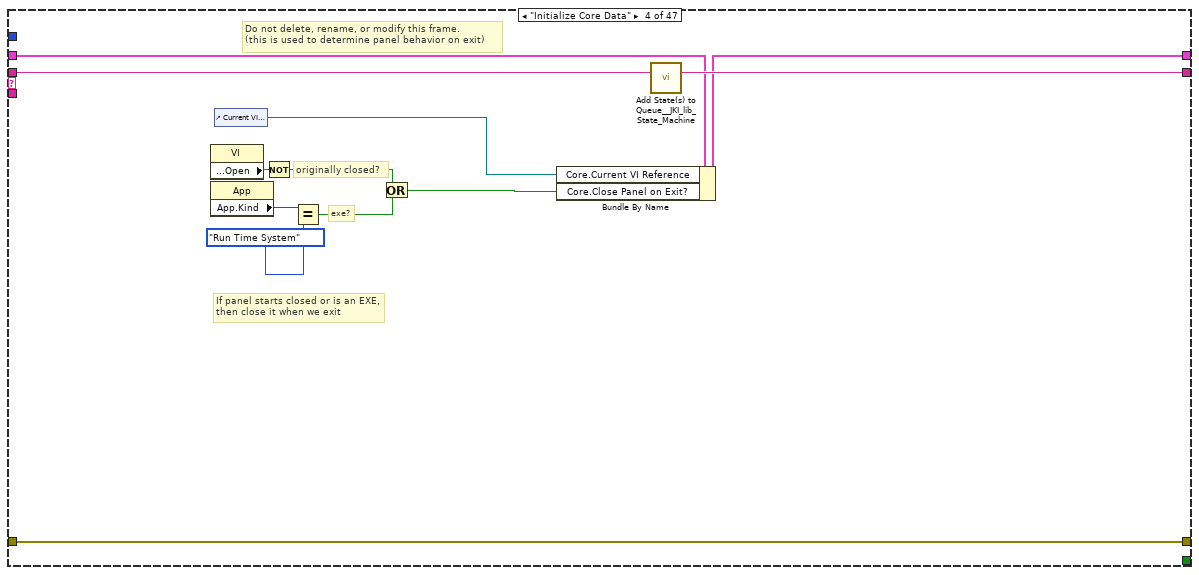
[diagram p20: hidden frame]
diagram:
  # "copy \"Example - Basic IPS-SA.vi\"\nValue (signaling) will execute event if value changes\nUse FGVs to remotely interact with this? (like lockin 4461?)\nwrite values to DSC. Which ones?\nHow to interact with both ITC and IPS? There is problem with \nMercury reference dissapearing"
  # "For instructions on how to use the JKI State Machine, examples and video tutorials, visit:\nhttp://jki.net/state-machine/\n\nJKI State Machine™\nhttp://jki.net/state-machine/\nCopyright (C) 2005-2015, JKI <info@jki.net>\nALL RIGHTS RESERVED"
  # "State Syntax:\nStateCategory: State >> Argument\nLine Terminator: Line feed\nExample:\nUI: Help >> About\n\nWhere \"UI\" is the state category\nWhere \"Help\" is the state\nWhere \"About\" is the argument\nOther Examples:\nApp Data: Initialize\nUI: Initialize\nHelp >> About\n\nCommenting:\nTo add a comment use \"//\" or \"#\" and all text to the right will be ignored\nCommenting Example:\nUI: Initialize // This initializes the UI\n# This whole line is a comment\n// Another comment line"
  # "copy this to create labels for wires"
  # "System_Label"
  n1 = call <vilib>:"Add State(s) to Queue__JKI_lib_State_Machine.vi"("State(s) in (\"\")"="Macro: Initialize") -> ("States Out"=w2:string)  [unwired: 14 in]
  n2 = while "JKI - String-Based Queued State Machine (Basic) v1.0" {
    shift-right: [w6] -> _
    shift-left: _ -> [w5]
    shift-right: [w9] -> _
    shift-left: _ -> [w3]
    shift-right: [w8] -> _
    shift-left: w2 -> [w10]
    stop <- w7 stop-if-true
    w4 = 10  # Timeout
    # "Template Copyright © 2015 JKI - http://jki.net/state-machine"
    n3 = call <vilib>:"Parse State Queue__JKI_lib_State_Machine.vi"("State Queue"=w10, "Error In (no error)"=w3) -> ("Remaining States"=w12:string, "Current State"=w13:string, "Arguments"=w11:string)  [unwired: 11 in]
    n4 = case shown="\"\", \"Event Structure\", \"Idle\"" w13 {
      selector: w13 -> [_ _ w119 _ _ _ _ _ _ _ _ _ _ _ _ _ _ _ _ _ _ _ _ _ _ _ _ _ _ _ _ _ _ _ _ _ _ _ _ _ _ _ _ _ _ _ _]
      tunnel: w12 -> [w20 w118 w123 w141 w158 w163 w167 w180 w186 w190 w200 w210 w221 w247 w254 w269 w273 w297 w346 w392 w434 w481 w504 w549 w590 w637 w678 w683 w705 w776 w813 w871 w887 w914 w918 w923 w963 w998 w1030 w1051 w1072 w1093 w1115 w1187 w1210 w1232 w1249]
      tunnel: w11 -> [_ _ _ _ _ _ _ _ _ _ _ w205 w215 _ _ _ _ _ _ _ _ _ _ _ _ _ _ _ _ _ _ _ _ _ _ _ _ _ _ _ _ _ _ _ _ _ _]
      tunnel: w5 -> [w16 w115 w121 w132 w144 w161 w164 _ w181 w187 w191 w208 w217 w244 w252 w267 w270 w292 w344 w391 w398 w441 w490 w547 w589 w636 w677 w680 w687 w744 w812 w828 w886 w913 w917 w920 w961 w987 w1025 w1040 w1061 w1082 w1101 w1172 w1197 w1215 w1236]
      tunnel: [w14 w116 w125 w138 errorcluster {"status"=FALSE, "code"=0, "source"=""} ("error out") w160 w165 w174 w182 w188 w195 w206 w218 w245 w251 w257 w271 w275 w306 w347 w395 w444 w491 w511 w556 w609 w644 w681 w690 w745 w784 w824 w884 w898 w916 w921 w933 w983 w1007 w1037 w1058 w1079 w1102 w1166 w1194 w1217 w1235] -> w9
      tunnel: [w19 w117 w122 w140 w157 w162 w166 w179 w185 w189 w199 w209 w220 w246 w253 w268 w272 w296 w345 w393 w435 w482 w505 w548 w591 w638 w679 w682 w706 w777 w814 w872 w888 w915 w919 w922 w964 w999 w1031 w1052 w1073 w1094 w1116 w1188 w1211 w1233 w1250] -> w8
      tunnel: [_ _ _ _ _ TRUE _ _ _ _ _ _ _ _ _ _ _ _ _ _ _ _ _ _ _ _ _ _ _ _ _ _ _ _ _ _ _ _ _ _ _ _ _ _ _ _ _] -> w7
      tunnel: [w18 w115 w121 w139 w143 w161 w164 w178 w181 w187 w192 w208 w217 w244 w252 w267 w270 w291 w344 w391 w398 w441 w490 w547 w589 w636 w677 w680 w686 w744 w812 w828 w886 w913 w917 w920 w961 w987 w1025 w1040 w1061 w1082 w1101 w1172 w1197 w1215 w1236] -> w6
      tunnel: w4 -> [w17 _ _ _ _ _ _ _ _ _ _ _ _ _ _ _ _ _ _ _ _ _ _ _ _ _ _ _ _ _ _ _ _ _ _ _ _ _ _ _ _ _ _ _ _ _ _]
      tunnel: w3 -> [w15 w116 w124 w138 w153 w160 w165 w174 w183 w188 w197 w207 w219 w245 w251 w259 w271 w284 w308 w358 w401 w443 w485 w513 w558 w596 w639 w681 w702 w775 w810 w861 w885 w892 w916 w921 w924 w993 w1022 w1046 w1067 w1088 w1103 w1182 w1198 w1218 w1234]
      frame "", "Event Structure", "Idle" {
        # "executes when the state queue is empty"
        n5 = event shown="[0] Timeout" {
          selector: _ -> [_ _ _ _ _ _ _ _ _ _ _ _ _ _]
          dyn-events: _ -> [_ _ _ _ _ _ _ _ _ _ _ _ _ _]
          timeout: w17 -> [_ _ _ _ _ _ _ _ _ _ _ _ _ _]
          tunnel: w20 -> [w39 w52 w58 w63 w67 w72 w77 w81 w87 w91 w96 w100 w108 w114]
          tunnel: [w38 w51 w57 w62 w66 w71 w76 w80 w86 w90 w95 w99 w107 w113] -> w19
          tunnel: [w21 w50 w54 w59 w64 w69 w74 w79 w84 w93 w98 w103 w105 w111] -> w18
          tunnel: w16 -> [w21 w50 w54 w59 w64 w69 w74 w79 w84 w93 w98 w103 w105 w111]
          tunnel: w15 -> [w24 w48 w55 w61 w68 w70 w75 w83 w85 w89 w94 w102 w106 w112]
          tunnel: [w23 w47 w55 w61 w68 w70 w75 w83 w85 w89 w94 w102 w106 w112] -> w14
          event Timeout {
            # "get remote"
            n6 = event-data() -> ()  [unwired: 1 in, 1 out]
            n7 = call <userlib>:"FGV_PSP - Mercury Remote.vi"("error in"=w24, "Function"=enum16{"write", "read"}."read") -> ("error out"=w23:errorcluster, "Remote"=w22:bool)  [unwired: 4 in]
            n8 = local write "Remote Mode"(w22) -> ()
            n9 = case shown="False" w22 {
              tunnel: ["Mercury: Idle\nMercury: IPS: Idle - 1\nMercury: IPS: Idle - 1a\nMercury: IPS: Idle - 2\nMercury: IPS: Idle - 3\nMercury: ITC: Idle" ("State(s) at Back (\"\")") "Mercury: Remote\nMercury: Idle\nMercury: IPS: Idle - 1\nMercury: IPS: Idle - 1a\nMercury: IPS: Idle - 2\nMercury: IPS: Idle - 3\nMercury: ITC: Idle" ("State(s) at Back (\"\")")] -> w27
              frame False {
              }
              frame True {
              }
            }
            n10 = while {
              shift-right: [w42] -> _
              shift-left: _ -> [w43]
              stop <- TRUE stop-if-true
              n11 = Get Date/Time In Seconds() -> (seconds since 1Jan1904=w42:timestamp)
              n12 = Subtract(x=w42, y=w43) -> (x-y=→"Iteration Time":dbl)
            }
            n13 = local read "Target Field (T)"() -> (w34:dbl)
            n14 = local read "Magnet Field (T)"() -> (w35:dbl)
            n15 = local read "Target Field Rate (T/min)"() -> (w37:dbl)
            n16 = local read "Power Supply Field (T)"() -> (w33:dbl)
            n17 = local read "SWITCH HEATER"() -> (w29:bool)
            n18 = local read "PS ON/OFF"() -> (w30:timestamp)
            n19 = local read "LPF ON"() -> (w32:timestamp)
            n20 = local read "Lambda"() -> (w26:bool)
            n21 = call "1820_Calculate_Sweep_Time.vi"("Power Supply Field (T)"=w33, "Target Field Rate (T/min)"=w37, "Magnet Field (T)"=w35, "Target Field (T)"=w34) -> ("ETA"=→"ETA":timestamp)  [unwired: 6 in, 1 out]
            n22 = call "1820_PS_ON_duration.vi"("SWITCH HEATER"=w29, "time stamp"=w30) -> ("PS Heat on (sec)"=→"PS Heat on or off (sec)":dbl)  [unwired: 9 in]
            n23 = call "1820_LPF_ON_duration.vi"("Lambda"=w26, "LPF ON"=w32) -> ("LPF on (sec)"=→"LPF on (sec)":dbl)  [unwired: 9 in]
            n24 = call <vilib>:"Add State(s) to Queue__JKI_lib_State_Machine.vi"("State(s) in Front (\"\")"=w27, "State(s) in (\"\")"=w39) -> ("States Out"=w38:string)  [unwired: 13 in]
          }
          event "Remote Mode": Value Change {
            n25 = event-data() -> ("NewVal"=w46:bool)  [unwired: 1 in, 5 out]
            n26 = call <userlib>:"FGV_PSP - Mercury Remote.vi"("error in"=w48, "Function"=enum16{"write", "read"}."write", "Remote"=w46) -> ("error out"=w47:errorcluster)  [unwired: 3 in, 1 out]
            n27 = call <vilib>:"Add State(s) to Queue__JKI_lib_State_Machine.vi"("State(s) in Front (\"\")"="Mercury: Remote", "State(s) in (\"\")"=w52) -> ("States Out"=w51:string)  [unwired: 13 in]
          }
          event "Hold": Value Change {
            n28 = event-data() -> ()  [unwired: 1 in, 6 out]
            n29 = call <vilib>:"Add State(s) to Queue__JKI_lib_State_Machine.vi"("State(s) in Front (\"\")"="Mercury: Hold" ("State(s) in Front (\"\")"), "State(s) in (\"\")"=w58) -> ("States Out"=w57:string)  [unwired: 13 in]
          }
          event "Clamp": Value Change {
            n30 = event-data() -> ()  [unwired: 1 in, 6 out]
            n31 = call <vilib>:"Add State(s) to Queue__JKI_lib_State_Machine.vi"("State(s) in Front (\"\")"="Mercury: Clamp" ("State(s) in Front (\"\")"), "State(s) in (\"\")"=w63) -> ("States Out"=w62:string)  [unwired: 13 in]
          }
          event "To Set": Value Change {
            n32 = event-data() -> ()  [unwired: 1 in, 6 out]
            n33 = call <vilib>:"Add State(s) to Queue__JKI_lib_State_Machine.vi"("State(s) in Front (\"\")"="Mercury: To Set" ("State(s) in Front (\"\")"), "State(s) in (\"\")"=w67) -> ("States Out"=w66:string)  [unwired: 13 in]
          }
          event "To Zero": Value Change {
            n34 = event-data() -> ()  [unwired: 1 in, 6 out]
            n35 = call <vilib>:"Add State(s) to Queue__JKI_lib_State_Machine.vi"("State(s) in Front (\"\")"="Mercury: To Zero" ("State(s) in Front (\"\")"), "State(s) in (\"\")"=w72) -> ("States Out"=w71:string)  [unwired: 13 in]
          }
          event "PS Heat": Value Change {
            n36 = event-data() -> ()  [unwired: 1 in, 6 out]
            n37 = call <vilib>:"Add State(s) to Queue__JKI_lib_State_Machine.vi"("State(s) in Front (\"\")"="Mercury: PS Heat" ("State(s) in Front (\"\")"), "State(s) in (\"\")"=w77) -> ("States Out"=w76:string)  [unwired: 13 in]
          }
          event "Send to IPS": Value Change {
            n38 = event-data() -> ()  [unwired: 1 in, 6 out]
            n39 = call <vilib>:"Add State(s) to Queue__JKI_lib_State_Machine.vi"("State(s) in Front (\"\")"="Mercury: Send To IPS" ("State(s) in Front (\"\")"), "State(s) in (\"\")"=w81) -> ("States Out"=w80:string)  [unwired: 13 in]
          }
          event "Lambda": Value Change {
            # "set lambda"
            n40 = event-data() -> ()  [unwired: 1 in, 6 out]
            n41 = call <vilib>:"Add State(s) to Queue__JKI_lib_State_Machine.vi"("State(s) in Front (\"\")"="Mercury: Lambda" ("State(s) in Front (\"\")"), "State(s) in (\"\")"=w87) -> ("States Out"=w86:string)  [unwired: 13 in]
          }
          event "Fast/Slow Fill": Value Change {
            n42 = event-data() -> ()  [unwired: 1 in, 6 out]
            n43 = call <vilib>:"Add State(s) to Queue__JKI_lib_State_Machine.vi"("State(s) in Front (\"\")"="Mercury: Fast/Slow Fill" ("State(s) in Front (\"\")"), "State(s) in (\"\")"=w91) -> ("States Out"=w90:string)  [unwired: 13 in]
          }
          event "Heater Current": Value Change {
            n44 = event-data() -> ()  [unwired: 1 in, 6 out]
            n45 = call <vilib>:"Add State(s) to Queue__JKI_lib_State_Machine.vi"("State(s) in Front (\"\")"="Mercury: Heater Current" ("State(s) in Front (\"\")"), "State(s) in (\"\")"=w96) -> ("States Out"=w95:string)  [unwired: 13 in]
          }
          event "Close Needle Valve", "Open Needle Valve": Value Change {
            n46 = event-data() -> ()  [unwired: 1 in, 6 out]
            n47 = call <vilib>:"Add State(s) to Queue__JKI_lib_State_Machine.vi"("State(s) in Front (\"\")"="Mercury: Needle Valve" ("State(s) in Front (\"\")"), "State(s) in (\"\")"=w100) -> ("States Out"=w99:string)  [unwired: 13 in]
          }
          event "OK": Value Change {
            # "Exit Button Value Change (pressed) Event\n(this executes Macro: Exit to terminate the VI)"
            n48 = event-data() -> ()  [unwired: 1 in, 1 out]
            n49 = call <vilib>:"Add State(s) to Queue__JKI_lib_State_Machine.vi"("State(s) in Front (\"\")"="Macro: Exit", "State(s) in (\"\")"=w108) -> ("States Out"=w107:string)  [unwired: 13 in]
          }
          event Panel Close? {
            # "Discard the event because we'll close the front panel ourselves in Macro: Exit"
            # "Close Panel button (pressed) Event\n(this executes Macro: Exit to terminate the VI)"
            n50 = event-data() -> ()  [unwired: 1 in, 1 out]
            n51 = call <vilib>:"Add State(s) to Queue__JKI_lib_State_Machine.vi"("State(s) in Front (\"\")"="Macro: Exit", "State(s) in (\"\")"=w114) -> ("States Out"=w113:string)  [unwired: 13 in]
            n52 = event-data("Discard?"=TRUE) -> ()  [unwired: 1 in, 1 out]
          }
        }
      }
      frame "---------- Core ----------" {
        # "Do not put any code in this frame.\n(it is a separator no-op)"
        n53 = call <vilib>:"Add State(s) to Queue__JKI_lib_State_Machine.vi"("State(s) in (\"\")"=w118) -> ("States Out"=w117:string)  [unwired: 14 in]
      }
      frame Default {
        w128 = 42 items=["No error", "Argument error", "Memory is full", "Out of zone", "End of file", "File already open", "Generic file I/O error", "File not found", "File permission error", "Disk is full", "Duplicate path", "Too many files open", "System feature not enabled", "Resource file not found", "Cannot add resource", "Resource not found", "Image not found", "Image memory error", "Pen does not exist", "Config type invalid", "Config token not found", "Config parse error", "Config memory error", "Bad external code format", "Bad external code offset", "External code not present", "Null window", "Destroy window error", "Null menu", "Print aborted", "Bad print record", "Print driver error", "Windows error during printing", "Memory error during printing", "Print dialog error", "Generic print error", "Invalid device refnum", "Device not found", "Device parameter error", "Device unit error", "Cannot open device", "Device call aborted", "Generic error", "Cancelled by user", "Object ID too low", "Object ID too high", "Object not in heap", "Unknown heap", "Unknown object (invalid DefProc)", "Unknown object (DefProc not in table)", "Message out of range", "Invalid (null) method", "Unknown message", "Manager call not supported", "Bad address", "Network operation in progress", "Network operation timed out", "Connection is busy", "Network attribute not supported", "Network error", "Address in use", "System out of memory", "Connection aborted", "Connection refused", "Not connected", "Already connected", "Connection closed", "Initialization error (interapplication manager)", "Bad occurrence", "Wait on unbound occurrence handler", "Occurrence queue overflow", "Datalog type conflict", "Unused", "Unrecognized type (interapplication manager)", "Memory corrupt", "Failed to make temporary DLL", "Old CIN version", "Drag socket not found", "Failed to load drop-object", "Failed to register OLE object", "Failed to release OLE object", "Format specifier type mismatch", "Unknown format specifier", "Too few format specifiers", "Too many format specifiers", "Scan failed", "Newer CIN version", "Error converting to variant", "Runtime menu error", "Password tampered", "Variant attribute not found", "Incompatible variant data type", "Event data is not available", "Event Store is not present", "Occurrence is not found", "Event Queue is not created", "Event info is not available", "Refnum passed is NULL", "Error retrieving Class GUID", "Error retrieving CoClass GUID", "Error retrieving TypeLib GUID.", "Bad built application magic bytes.", "Specific driver is different from the specific driver associated with the Logical Name.", "There is no session opened to the class driver.", "Max Error", "MAX - Error with config objects", "MAX - Error loading configuration", "MAX - Group not supported"]
        # "Current State"
        # "Do not delete, rename, or modify this frame.\n(this is used to capture unhandled states and typos)"
        # "Handle mistyped state name (developer tool)"
        n54 = Format Into String(format string="Software Exception: Unhandled State \"%s\"." ("message"), error in=w124, w119) -> (resulting string=w127:string, error out=w126:errorcluster)  [unwired: 1 in]
        n55 = call <vilib>:"Error Cluster From Error Code.vi"("show call chain? (False)"=TRUE, "error in (no error)"=w126, "error message (\"\")"=w127, "error code (0)"=w128) -> ("error out"=w125:errorcluster)  [unwired: 5 in]
        n56 = call <vilib>:"Add State(s) to Queue__JKI_lib_State_Machine.vi"("State(s) in (\"\")"=w123) -> ("States Out"=w122:string)  [unwired: 14 in]
      }
      frame "Initialize Core Data" {
        # "Do not delete, rename, or modify this frame.\n(this is used to determine panel behavior on exit)"
        # "originally closed?"
        # "exe?"
        # "If panel starts closed or is an EXE, then close it when we exit"
        n57 = property class="VI"() -> ("Front Panel.Open"=w137:bool)  [unwired: 2 in, 2 out]
        n58 = property class="App"() -> ("App.Kind"=w136:T26)  [unwired: 2 in, 2 out]
        n59 = control-ref of="Current VI Reference"() -> (w130:refnum<vi>)
        n60 = Not(x=w137) -> (.not. x?=w134:bool)
        n61 = Equal?(x=w136, y=T26."Run Time System" ("Application:Kind")) -> (x = y?=w133:bool)
        n62 = Or(x=w134, y=w133) -> (x .or. y?=w131:bool)
        n63 = Bundle By Name(cluster=w132, "Core.Current VI Reference"=w130, "Core.Close Panel on Exit?"=w131) -> (w139:T39)
        n64 = call <vilib>:"Add State(s) to Queue__JKI_lib_State_Machine.vi"("State(s) in (\"\")"=w141) -> ("States Out"=w140:string)  [unwired: 14 in]
      }
      frame "Error Handler" {
        w152 = i32[] [-1950679035, -1950678943]  # Error Codes to Filter
        # "Unhandled Error -- Display it"
        # "Handle any errors here.\nYou can also output any states to clean-up after errors occur"
        # "Clear error"
        n65 = call-poly <userlib>:"Filter Error Codes__ogtk.vi"("Error In"=w153, "Error Codes to Filter"=w152) -> ("Error Out"=w154:errorcluster, "Filtered Error Details"=w151:T40)  [unwired: 7 in, 1 out]
        n66 = Unbundle(w151) -> ("code"=w149:i32, "source"=w150:string)
        n67 = Get Date/Time In Seconds() -> (seconds since 1Jan1904=w148:timestamp)
        n68 = Unbundle By Name(w144) -> ("Error Log"=w146:T25)
        n69 = Bundle By Name(cluster=T27 {"time"=timestamp(0 s since 1904-01-01), "code"=0, "source"=""} ("output cluster"), "time"=w148, "code"=w149, "source"=w150) -> (w145:T27)
        n70 = Build Array (concatenate)(w146, w145) -> (w142:T25)
        "Error List" <- w142
        n71 = Bundle By Name(cluster=w144, "Error Log"=w142) -> (w143:T39)
        n72 = call <vilib>:"General Error Handler.vi"("error in (no error)"=w154) -> ()  [unwired: 10 in, 5 out]
        n73 = call <vilib>:"Add State(s) to Queue__JKI_lib_State_Machine.vi"("State(s) in Front (\"\")"="/* Post Error States", "State(s) in (\"\")"=w158) -> ("States Out"=w157:string)  [unwired: 13 in]
      }
      frame "Exit" {
        # "Do not put any code in this frame.\n(No errors that occur here will be handled.)"
        n74 = call <vilib>:"Add State(s) to Queue__JKI_lib_State_Machine.vi"("State(s) in (\"\")"=w163) -> ("States Out"=w162:string)  [unwired: 14 in]
      }
      frame "---------- Data ----------" {
        # "Do not put any code in this frame.\n(It is a separator no-op. You can make a copy of this frame to create a new Data frame)"
        n75 = call <vilib>:"Add State(s) to Queue__JKI_lib_State_Machine.vi"("State(s) in (\"\")"=w167) -> ("States Out"=w166:string)  [unwired: 14 in]
      }
      frame "Data: Initialize" {
        w168 = bool[] [FALSE, FALSE, FALSE, FALSE, FALSE, FALSE, FALSE, FALSE]  # LEDs
        w169 = 0  # counter
        w171 = TRUE  # read ITC T?
        w172 = T36 {"Comms"="", "Device ID"=[], "Comms Layer"=enum."Ethernet TCP/IP", "Command"="", "Query reference"=refnum}  # Mercury ITC Ref
        w173 = T25 []  # Error Log
        w175 = TRUE  # sentinel
        w176 = T36 {"Comms"="", "Device ID"=[], "Comms Layer"=enum."Ethernet TCP/IP", "Command"="", "Query reference"=refnum}  # Mercury IPS Ref
        w177 = T41 {"Current VI Reference"=refnum, "Close Panel on Exit?"=FALSE}  # Core
        # "read FGV in timeout"
        # "do not delete - used by framework"
        # "Data names and types of shift register data are defined by this bundle."
        # "Initialize the shift-register data, here.\n(data names are defined by what you wire into the bundle function)"
        n76 = call <vilib>:"Add State(s) to Queue__JKI_lib_State_Machine.vi"("State(s) in (\"\")"=w180) -> ("States Out"=w179:string)  [unwired: 14 in]
        n77 = call "MercuryStateHistory.vi"("initialize?"=TRUE) -> ()  [unwired: 9 in, 2 out]
        n78 = Bundle("Core"=w177, "Mercury ITC Ref"=w172, "Mercury IPS Ref"=w176, "sentinel"=w175, "Error Log"=w173, "read ITC T?"=w171, "counter"=w169, "LEDs"=w168) -> (w178:T39)  [unwired: 1 in]
      }
      frame "Data: Cleanup" {
        # "Cleanup any data and references, here.\n(this is called automatically, by the Macro: Exit)"
        n79 = Unbundle By Name(w181) -> ("Core.Current VI Reference"=w184:refnum<vi>)
        n80 = Close Reference(reference=w184, error in (no error)=w183) -> (error out=w182:errorcluster)
        n81 = call <vilib>:"Add State(s) to Queue__JKI_lib_State_Machine.vi"("State(s) in (\"\")"=w186) -> ("States Out"=w185:string)  [unwired: 14 in]
      }
      frame "---------- UI ----------" {
        # "Do not put any code in this frame.\n(It is a separator no-op. You can make a copy of this frame to create a new UI frame)"
        n82 = call <vilib>:"Add State(s) to Queue__JKI_lib_State_Machine.vi"("State(s) in (\"\")"=w190) -> ("States Out"=w189:string)  [unwired: 14 in]
      }
      frame "UI: Initialize" {
        w193 = bool[] [TRUE, FALSE, TRUE, FALSE, TRUE, FALSE, TRUE, FALSE] ("LEDs")
        w196 = FALSE
        # "start in local mode"
        # "Initialize the User Interface, here.\n(this is called automatically, by the Macro: Init)"
        n83 = disable-structure shown="Enabled" {
          frame Disabled {
            n84 = Open Application Reference() -> (0:w202:errorcluster, 3:w201:refnum<vi>)  [unwired: 4 in]
            n85 = Open VI Reference(vi path=path "") -> ()  [unwired: 5 in, 2 out]
            n86 = property class="App"(reference=w201, error in=w202, "WebSrvr.Active"=TRUE ("Web Server:Server Active")) -> ()  [unwired: 2 out]
            n87 = call "MNK_Dashboard_v2.vi"() -> ()  [unwired: 12 in]
          }
          frame Enabled {
          }
        }
        n88 = call <userlib>:"Fit VI window to Largest Dec__ogtk.vi"("error in (no error)"=w197) -> ("error out"=w194:errorcluster)  [unwired: 5 in, 1 out]
        n89 = local write "Remote Mode"(w196) -> ()
        n90 = call <vilib>:"Add State(s) to Queue__JKI_lib_State_Machine.vi"("State(s) in (\"\")"=w200) -> ("States Out"=w199:string)  [unwired: 14 in]
        n91 = call <userlib>:"FGV_PSP - Mercury Remote.vi"("error in"=w194, "Remote"=w196) -> ("error out"=w195:errorcluster)  [unwired: 4 in, 1 out]
        n92 = local write "LEDs"(w193) -> ()
        n93 = Bundle By Name(cluster=w191, "LEDs"=w193) -> (w192:T39)
        "Magnet Status 2" <- "" ("Magnet Status 2")
      }
      frame "UI: Cursor Set" {
        # "Argument"
        # "Set and Unset Cursor Busy.\n(Usage: \"UI: Cursor Set >> Busy|Idle\")"
        n94 = case shown="\"Idle\", Default" w205 {
          tunnel: w207 -> [w212 w214]
          tunnel: [w211 w213] -> w206
          frame "Idle", Default {
            n95 = call <vilib>:"Unset Busy.vi"("error in (no error)"=w212) -> ("error out"=w211:errorcluster)  [unwired: 10 in]
          }
          frame "Busy" {
            n96 = call <vilib>:"Set Busy.vi"("error in (no error)"=w214) -> ("error out"=w213:errorcluster)  [unwired: 9 in, 1 out]
          }
        }
        n97 = call <vilib>:"Add State(s) to Queue__JKI_lib_State_Machine.vi"("State(s) in (\"\")"=w210) -> ("States Out"=w209:string)  [unwired: 14 in]
      }
      frame "UI: Front Panel State" {
        # "Argument"
        # "Set Front Panel Open or Closed\n(Usage: \"UI: Front Panel State >> Open|Close\")"
        n98 = Unbundle By Name(w217) -> ("Core.Current VI Reference"=w216:refnum<vi>)
        n99 = case shown="\"Open\", Default" w215 {
          tunnel: w219 -> [w225 w238]
          tunnel: [w227 w239] -> w218
          tunnel: w216 -> [w226 w236]
          frame "Open", Default {
            n100 = property class="VI"(reference=w226, error in=w225) -> (reference out=w223:refnum<vi>, error out=w224:errorcluster, "Front Panel.Open"=w222:bool)
            n101 = case shown="True" w222 {
              tunnel: [w230 w233] -> w227
              tunnel: w224 -> [w229 w233]
              tunnel: w223 -> [w228 _]
              frame False {
                n102 = invoke class="VI" method="FP.Open"(reference=w228, error in=w229, "Activate"=TRUE, "State"=T28."Standard") -> (error out=w230:errorcluster)  [unwired: 1 in, 4 out]
              }
              frame True {
              }
            }
          }
          frame "Close" {
            n103 = property class="VI"(reference=w236, error in=w238) -> (reference out=w235:refnum<vi>, error out=w237:errorcluster, "Front Panel.Open"=w234:bool)
            n104 = case shown="True" w234 {
              tunnel: [w240 w243] -> w239
              tunnel: w237 -> [w240 w242]
              tunnel: w235 -> [_ w241]
              frame False {
              }
              frame True {
                n105 = invoke class="VI" method="FP.Close"(reference=w241, error in=w242) -> (error out=w243:errorcluster)  [unwired: 1 in, 2 out]
              }
            }
          }
        }
        n106 = call <vilib>:"Add State(s) to Queue__JKI_lib_State_Machine.vi"("State(s) in (\"\")"=w221) -> ("States Out"=w220:string)  [unwired: 14 in]
      }
      frame "---------- Macro ----------" {
        # "Do not put any code in this frame.\n(It is a separator no-op. You can make a copy of this frame to create a new Macro frame)"
        n107 = call <vilib>:"Add State(s) to Queue__JKI_lib_State_Machine.vi"("State(s) in (\"\")"=w247) -> ("States Out"=w246:string)  [unwired: 14 in]
      }
      frame "Macro: Initialize" {
        w250 = "Data: Initialize\nInitialize Core Data\nUI: Initialize\nUI: Front Panel State >> Open"  # Data: Initialize Initialize Core Data UI: Initialize UI: Front Panel State >> Open
        # "Initialization Macro\n(This is called once, when the VI starts)"
        n108 = call <vilib>:"Add State(s) to Queue__JKI_lib_State_Machine.vi"("State(s) in Front (\"\")"=w250, "State(s) at Back (\"\")"="Mercury: Initialize") -> ("States Out"=w249:string)  [unwired: 13 in]
        n109 = call <vilib>:"Add State(s) to Queue__JKI_lib_State_Machine.vi"("State(s) in Front (\"\")"=w249, "State(s) in (\"\")"=w254) -> ("States Out"=w253:string)  [unwired: 13 in]
      }
      frame "Macro: Exit" {
        # "Exit Macro\n(This is called once, when the VI exits)"
        n110 = Unbundle By Name(w267) -> ("Core.Close Panel on Exit?"=w266:bool, "Mercury ITC Ref"=w255:T36, "Mercury IPS Ref"=w256:T36)
        n111 = call <instrlib>:"Close.vi"("error in (no error)"=w259, "Mercury Reference"=w256) -> ("error out"=w258:errorcluster)  [unwired: 9 out]
        n112 = call <instrlib>:"Close.vi"("error in (no error)"=w258, "Mercury Reference"=w255) -> ("error out"=w260:errorcluster)  [unwired: 9 out]
        n113 = call <vilib>:"Simple Error Handler.vi"("error in (no error)"=w260) -> ("error out"=w257:errorcluster)  [unwired: 1 in, 7 out]
        n114 = Select(t="UI: Front Panel State >> Close", s=w266, f="") -> (s? t:f=w263:string)
        n115 = call <vilib>:"Add State(s) to Queue__JKI_lib_State_Machine.vi"("State(s) in (\"\")"=w263, "State(s) at Back (\"\")"="Data: Cleanup\nExit") -> ("States Out"=w261:string)  [unwired: 13 in]
        n116 = call <vilib>:"Add State(s) to Queue__JKI_lib_State_Machine.vi"("State(s) in Front (\"\")"=w261, "State(s) in (\"\")"=w269) -> ("States Out"=w268:string)  [unwired: 13 in]
      }
      frame "---------- Mercury: Query ----------" {
        n117 = call <vilib>:"Add State(s) to Queue__JKI_lib_State_Machine.vi"("State(s) in (\"\")"=w273) -> ("States Out"=w272:string)  [unwired: 14 in]
      }
      frame "Mercury: Initialize" {
        w283 = Comms_Transport_Layer."Ethernet TCP/IP" ("Comms Layer")
        n118 = call-poly <instrlib>:"Open.vi"("Clear Previous Connections (False)"=TRUE ("Clear Previous Connections (True)"), "ID Query (True)"=TRUE, "IP Address"="ITC IP Address", "error in (no error)"=w284, "Comms Layer"=w283) -> ("error out"=w278:errorcluster, "# of Instruments"=→"# of Instruments":i32, "Serial Number(s)"=→"Serial Number(s)":string[], "Mercury Reference Out"=w279:T36, "S/W Version(s)"=→"S/W Version(s)":string[])  [unwired: 2 in]
        n119 = call-poly <instrlib>:"Open.vi"("Clear Previous Connections (False)"=FALSE ("Clear Previous Connections (True)"), "ID Query (True)"=TRUE, "IP Address"="IPS IP Address", "error in (no error)"=w278, "Comms Layer"=w283) -> ("error out"=w275:errorcluster, "# of Instruments"=→"# of Instruments 2":i32, "Serial Number(s)"=→"Serial Number(s) 2":string[], "Mercury Reference Out"=w277:T36, "S/W Version(s)"=→"S/W Version(s) 2":string[])  [unwired: 2 in]
        n120 = case shown="No Error" w275 {
          tunnel: ["Mercury: Query ITC: System\nMercury: Query IPS: System\nMercury: Query ITC: Temperature\nMercury: Query ITC: Heater\nMercury: Query ITC: Aux\nMercury: Query ITC: Pressure\nMercury: Query IPS: LVL\nMercury: Query IPS: Temperature\nMercury: Query IPS: Magnet" ("State(s) at Back (\"\")") "Error Handler\nMacro: Exit" ("State(s) at Back (\"\")")] -> w276
          tunnel: [bool[] [TRUE, FALSE, TRUE, FALSE, TRUE, FALSE, TRUE, FALSE] ("LEDs") w301] -> w274
          frame No Error {
            n121 = local write "LEDs"(bool[] [TRUE, TRUE, TRUE, TRUE, TRUE, TRUE, TRUE, TRUE] ("LEDs")) -> ()
          }
          frame Error {
            w301 = bool[] [FALSE, FALSE, FALSE, FALSE, FALSE, FALSE, FALSE, FALSE] ("LEDs")
            n122 = local write "LEDs"(w301) -> ()
          }
        }
        n123 = Bundle By Name(cluster=w292, "Mercury ITC Ref"=w279, "Mercury IPS Ref"=w277, "LEDs"=w274) -> (w291:T39)
        n124 = call <vilib>:"Add State(s) to Queue__JKI_lib_State_Machine.vi"("State(s) in Front (\"\")"=w276, "State(s) in (\"\")"=w297) -> ("States Out"=w296:string)  [unwired: 13 in]
      }
      frame "Mercury: Query ITC: System" {
        n125 = Unbundle By Name(w344) -> ("Mercury ITC Ref"=w304:T36)
        n126 = call-poly <instrlib>:"Configuration (Read).vi"("error in"=w308, "Mercury Reference In"=w304) -> ("error out"=w340:errorcluster, "Devices"=→"ITC Devices":string[], "Mercury Reference Out"=w341:T36)  [unwired: 1 in, 6 out]
        n127 = call-poly <instrlib>:"Configuration (Read).vi"("error in"=w340, "Mercury Reference In"=w341) -> ("error out"=w333:errorcluster, "Automatic Dimming"=→"Automatic Dimming":string, "Mercury Reference Out"=w334:T36)  [unwired: 1 in, 6 out]
        n128 = call-poly <instrlib>:"Configuration (Read).vi"("error in"=w333, "Mercury Reference In"=w334) -> ("error out"=w336:errorcluster, "Dimming Time"=→"Dimming Time":string, "Mercury Reference Out"=w335:T36)  [unwired: 1 in, 6 out]
        n129 = call-poly <instrlib>:"Configuration (Read).vi"("error in"=w336, "Mercury Reference In"=w335) -> ("error out"=w342:errorcluster, "Display Brightness"=→"Display Brightness":string, "Mercury Reference Out"=w343:T36)  [unwired: 1 in, 6 out]
        n130 = call-poly <instrlib>:"Configuration (Read).vi"("error in"=w342, "Mercury Reference In"=w343) -> ("error out"=w327:errorcluster, "Date"=→"Date":string, "Mercury Reference Out"=w326:T36)  [unwired: 1 in, 6 out]
        n131 = call-poly <instrlib>:"Configuration (Read).vi"("error in"=w327, "Mercury Reference In"=w326) -> ("error out"=w329:errorcluster, "Time"=→"Time":string, "Mercury Reference Out"=w328:T36)  [unwired: 1 in, 6 out]
        n132 = call-poly <instrlib>:"Configuration (Read).vi"("error in"=w329, "Mercury Reference In"=w328) -> ("error out"=w307:errorcluster, "time stamp"=→"time stamp":timestamp, "Mercury Reference Out"=w305:T36)  [unwired: 1 in, 6 out]
        n133 = call-poly <instrlib>:"Configuration (Read).vi"("error in"=w307, "Mercury Reference In"=w305) -> ("error out"=w325:errorcluster, "Hardware Version"=→"Hardware Version":string, "Mercury Reference Out"=w324:T36)  [unwired: 1 in, 6 out]
        n134 = call-poly <instrlib>:"Configuration (Read).vi"("error in"=w325, "Mercury Reference In"=w324) -> ("error out"=w323:errorcluster, "Firmware Version"=→"Firmware Version":string, "Mercury Reference Out"=w322:T36)  [unwired: 1 in, 6 out]
        n135 = call-poly <instrlib>:"Configuration (Read).vi"("error in"=w323, "Mercury Reference In"=w322) -> ("error out"=w310:errorcluster, "Serial Number"=→"Serial Number":string, "Mercury Reference Out"=w309:T36)  [unwired: 1 in, 6 out]
        n136 = call-poly <instrlib>:"Configuration (Read).vi"("error in"=w310, "Mercury Reference In"=w309) -> ("error out"=w316:errorcluster, "Free Space"=→"Free Space":i32, "Mercury Reference Out"=w315:T36)  [unwired: 1 in, 6 out]
        n137 = call-poly <instrlib>:"Configuration (Read).vi"("error in"=w316, "Mercury Reference In"=w315) -> ("error out"=w312:errorcluster, "Mode"=→"String":T32, "Mercury Reference Out"=w313:T36)  [unwired: 1 in, 6 out]
        n138 = Get Date/Time In Seconds() -> (seconds since 1Jan1904=w321:timestamp)
        n139 = call-poly <instrlib>:"Configuration (Set).vi"("error in"=w312, "time stamp"=w321, "Mercury Reference In"=w313) -> ("error out"=w306:errorcluster, "Response"=→"Set Date Response":T35)  [unwired: 1 in, 6 out]
        n140 = call <vilib>:"Add State(s) to Queue__JKI_lib_State_Machine.vi"("State(s) in (\"\")"=w346) -> ("States Out"=w345:string)  [unwired: 14 in]
      }
      frame "Mercury: Query ITC: Temperature" {
        # "Temperature"
        n141 = Unbundle By Name(w391) -> ("Mercury ITC Ref"=w353:T36)
        n142 = local read "ITC Devices"() -> (w352:string[])
        n143 = Index Array(array=w352, index=3) -> (element=w354:string)
        n144 = call-poly <instrlib>:"Open.vi"("error in (no error)"=w358, "Device Identifier"=w354, "Mercury Reference In"=w353) -> ("error out"=w370:errorcluster, "Mercury Reference Out"=w371:T36)  [unwired: 7 out]
        n145 = call-poly <instrlib>:"Configuration (Read).vi"("error in"=w370, "Mercury Reference In"=w371) -> ("error out"=w362:errorcluster, "Serial Number"=→"Temp S/N":string, "Mercury Reference Out"=w361:T36)  [unwired: 1 in, 6 out]
        n146 = call-poly <instrlib>:"Configuration (Read).vi"("error in"=w362, "Mercury Reference In"=w361) -> ("error out"=w364:errorcluster, "Nickname"=→"T Nickname":string, "Mercury Reference Out"=w363:T36)  [unwired: 1 in, 6 out]
        n147 = call-poly <instrlib>:"Configuration (Read).vi"("error in"=w364, "Mercury Reference In"=w363) -> ("error out"=w367:errorcluster, "Unit"=→"Unit":T3, "Excitation Magnitude"=→"Excitation Magnitude":dbl, "Mercury Reference Out"=w366:T36)  [unwired: 1 in, 5 out]
        n148 = call-poly <instrlib>:"Configuration (Read).vi"("error in"=w367, "Mercury Reference In"=w366) -> ("error out"=w357:errorcluster, "Sensor Type"=→"Sensor Type":T42, "Mercury Reference Out"=w355:T36)  [unwired: 1 in, 6 out]
        n149 = call-poly <instrlib>:"Configuration (Read).vi"("error in"=w357, "Mercury Reference In"=w355) -> ("error out"=w373:errorcluster, "Excitation Type"=→"Excitation Type":T7, "Mercury Reference Out"=w374:T36)  [unwired: 1 in, 6 out]
        n150 = call-poly <instrlib>:"Configuration (Read).vi"("error in"=w373, "Mercury Reference In"=w374) -> ("error out"=w375:errorcluster, "Unit"=→"H Unit":T3, "Hot Limit"=→"Hot Limit":dbl, "Mercury Reference Out"=w376:T36)  [unwired: 1 in, 5 out]
        n151 = call-poly <instrlib>:"Configuration (Read).vi"("error in"=w375, "Mercury Reference In"=w376) -> ("error out"=w382:errorcluster, "Unit"=→"C Unit":T3, "Cold Limit"=→"Cold Limit":dbl, "Mercury Reference Out"=w381:T36)  [unwired: 1 in, 5 out]
        n152 = call-poly <instrlib>:"Signals (Read).vi"("error in"=w382, "Mercury Reference In"=w381) -> ("error out"=w386:errorcluster, "Unit"=→"V Unit":T3, "Voltage"=→"Voltage":dbl, "Mercury Reference Out"=w385:T36)  [unwired: 1 in, 5 out]
        n153 = call-poly <instrlib>:"Signals (Read).vi"("error in"=w386, "Mercury Reference In"=w385) -> ("error out"=w387:errorcluster, "Unit"=→"T Unit":T3, "Temperature"=→"Temperature":dbl, "Mercury Reference Out"=w390:T36)  [unwired: 1 in, 5 out]
        n154 = call-poly <instrlib>:"Configuration (Read).vi"("error in"=w387, "Mercury Reference In"=w390) -> ("error out"=w347:errorcluster, "Device Details"=w348:T43)  [unwired: 1 in, 7 out]
        n155 = Unbundle By Name(w348) -> ("Manufacturing"=→"ITC Manufacturing":T8, "Excitation"=→"ITC Excitation":T6, "Calibration"=→"ITC Calibration":T4)
        n156 = call <vilib>:"Add State(s) to Queue__JKI_lib_State_Machine.vi"("State(s) in (\"\")"=w392) -> ("States Out"=w393:string)  [unwired: 14 in]
      }
      frame "Mercury: Query ITC: Heater" {
        # "Heater"
        n157 = Unbundle By Name(w398) -> ("Mercury ITC Ref"=w397:T36)
        n158 = local read "ITC Devices"() -> (w399:string[])
        n159 = Index Array(array=w399, index=2) -> (element=w394:string)
        n160 = call-poly <instrlib>:"Open.vi"("error in (no error)"=w401, "Device Identifier"=w394, "Mercury Reference In"=w397) -> ("error out"=w404:errorcluster, "Mercury Reference Out"=w403:T36)  [unwired: 7 out]
        n161 = call-poly <instrlib>:"Configuration (Read).vi"("error in"=w404, "Mercury Reference In"=w403) -> ("error out"=w411:errorcluster, "Device Details"=→"Heater Device Settings":T9, "Mercury Reference Out"=w410:T36)  [unwired: 1 in, 6 out]
        n162 = call-poly <instrlib>:"Configuration (Read).vi"("error in"=w411, "Mercury Reference In"=w410) -> ("error out"=w413:errorcluster, "Nickname"=→"Htr Nickname":string, "Mercury Reference Out"=w412:T36)  [unwired: 1 in, 6 out]
        n163 = call-poly <instrlib>:"Configuration (Read).vi"("error in"=w413, "Mercury Reference In"=w412) -> ("error out"=w406:errorcluster, "Serial Number"=→"Htr S/N":string, "Mercury Reference Out"=w405:T36)  [unwired: 1 in, 6 out]
        n164 = call-poly <instrlib>:"Configuration (Read).vi"("error in"=w406, "Mercury Reference In"=w405) -> ("error out"=w402:errorcluster, "Unit"=→"Volt Unit":T3, "Voltage Limit"=→"Htr Voltage Limit":dbl, "Mercury Reference Out"=w396:T36)  [unwired: 1 in, 5 out]
        n165 = call-poly <instrlib>:"Configuration (Read).vi"("error in"=w402, "Mercury Reference In"=w396) -> ("error out"=w416:errorcluster, "Unit"=→"Res Unit":T3, "Nominal Resistance"=→"Htr Resistance":dbl, "Mercury Reference Out"=w417:T36)  [unwired: 1 in, 5 out]
        n166 = call-poly <instrlib>:"Configuration (Read).vi"("error in"=w416, "Mercury Reference In"=w417) -> ("error out"=w423:errorcluster, "Unit"=→"Power Unit":T3, "Maximum Power"=→"Maximum Power":dbl, "Mercury Reference Out"=w422:T36)  [unwired: 1 in, 5 out]
        n167 = call-poly <instrlib>:"Signals (Read).vi"("error in"=w423, "Mercury Reference In"=w422) -> ("error out"=w425:errorcluster, "Unit"=→"Htr V Unit":T3, "Voltage"=→"Htr Voltage":dbl, "Mercury Reference Out"=w424:T36)  [unwired: 1 in, 5 out]
        n168 = call-poly <instrlib>:"Signals (Read).vi"("error in"=w425, "Mercury Reference In"=w424) -> ("error out"=w427:errorcluster, "Unit"=→"Htr P Unit":T3, "Power"=→"Htr Power":dbl, "Mercury Reference Out"=w426:T36)  [unwired: 1 in, 5 out]
        n169 = call-poly <instrlib>:"Signals (Read).vi"("error in"=w427, "Mercury Reference In"=w426) -> ("error out"=w395:errorcluster, "Unit"=→"Htr C Unit":T3, "Current"=→"Htr Current":dbl)  [unwired: 1 in, 6 out]
        n170 = call <vilib>:"Add State(s) to Queue__JKI_lib_State_Machine.vi"("State(s) in (\"\")"=w434) -> ("States Out"=w435:string)  [unwired: 14 in]
      }
      frame "Mercury: Query ITC: Aux" {
        # "Auxiliary"
        n171 = Unbundle By Name(w441) -> ("Mercury ITC Ref"=w436:T36)
        n172 = local read "ITC Devices"() -> (w439:string[])
        n173 = Index Array(array=w439, index=0) -> (element=w437:string)
        n174 = call-poly <instrlib>:"Open.vi"("error in (no error)"=w443, "Device Identifier"=w437, "Mercury Reference In"=w436) -> ("error out"=w463:errorcluster, "Mercury Reference Out"=w464:T36)  [unwired: 7 out]
        n175 = call-poly <instrlib>:"Configuration (Read).vi"("error in"=w463, "Mercury Reference In"=w464) -> ("error out"=w467:errorcluster, "Auxiliary Device Details"=→"Auxiliary Device Details":T12, "Mercury Reference Out"=w466:T36)  [unwired: 1 in, 6 out]
        n176 = call-poly <instrlib>:"Configuration (Read).vi"("error in"=w467, "Mercury Reference In"=w466) -> ("error out"=w470:errorcluster, "Serial Number"=→"Aux S/N":string, "Mercury Reference Out"=w469:T36)  [unwired: 1 in, 6 out]
        n177 = call-poly <instrlib>:"Configuration (Read).vi"("error in"=w470, "Mercury Reference In"=w469) -> ("error out"=w472:errorcluster, "Unit"=→"Unit 2":T3, "Min Flow"=→"Min Flow":dbl, "Mercury Reference Out"=w471:T36)  [unwired: 1 in, 5 out]
        n178 = call-poly <instrlib>:"Configuration (Read).vi"("error in"=w472, "Mercury Reference In"=w471) -> ("error out"=w474:errorcluster, "Unit"=→"Unit 3":T3, "Scaling Factor"=→"Scaling Factor":dbl, "Mercury Reference Out"=w473:T36)  [unwired: 1 in, 5 out]
        n179 = call-poly <instrlib>:"Configuration (Read).vi"("error in"=w474, "Mercury Reference In"=w473) -> ("error out"=w442:errorcluster, "Unit"=→"Unit 4":T3, "Temp Err"=→"Temp Err":dbl, "Mercury Reference Out"=w438:T36)  [unwired: 1 in, 5 out]
        n180 = call-poly <instrlib>:"Configuration (Read).vi"("error in"=w442, "Mercury Reference In"=w438) -> ("error out"=w446:errorcluster, "Unit"=→"Unit 5":T3, "Temp V Err"=→"Temp V Err":dbl, "Mercury Reference Out"=w445:T36)  [unwired: 1 in, 5 out]
        n181 = call-poly <instrlib>:"Configuration (Read).vi"("error in"=w446, "Mercury Reference In"=w445) -> ("error out"=w448:errorcluster, "Unit"=→"Unit 6":T3, "Gear"=→"Gear":u32, "Mercury Reference Out"=w447:T36)  [unwired: 1 in, 5 out]
        n182 = call-poly <instrlib>:"Configuration (Read).vi"("error in"=w448, "Mercury Reference In"=w447) -> ("error out"=w456:errorcluster, "Unit"=→"Unit 7":T3, "Speed"=→"Speed":u32, "Mercury Reference Out"=w455:T36)  [unwired: 1 in, 5 out]
        n183 = call-poly <instrlib>:"Signals (Read).vi"("error in"=w456, "Mercury Reference In"=w455) -> ("error out"=w458:errorcluster, "Unit"=→"Unit":T3, "Position"=→"Position":u32, "Mercury Reference Out"=w457:T36)  [unwired: 1 in, 5 out]
        n184 = call-poly <instrlib>:"Signals (Read).vi"("error in"=w458, "Mercury Reference In"=w457) -> ("error out"=w444:errorcluster, "Unit"=→"Unit":T3, "% Open"=→"% Open":dbl)  [unwired: 1 in, 6 out]
        n185 = call <vilib>:"Add State(s) to Queue__JKI_lib_State_Machine.vi"("State(s) in (\"\")"=w481) -> ("States Out"=w482:string)  [unwired: 14 in]
      }
      frame "Mercury: Query ITC: Pressure" {
        # "Pressure"
        n186 = Unbundle By Name(w490) -> ("Mercury ITC Ref"=w487:T36)
        n187 = local read "ITC Devices"() -> (w489:string[])
        n188 = Index Array(array=w489, index=1) -> (element=w486:string)
        n189 = call-poly <instrlib>:"Open.vi"("error in (no error)"=w485, "Device Identifier"=w486, "Mercury Reference In"=w487) -> ("error out"=w493:errorcluster, "Mercury Reference Out"=w494:T36)  [unwired: 7 out]
        n190 = call-poly <instrlib>:"Configuration (Read).vi"("error in"=w493, "Mercury Reference In"=w494) -> ("error out"=w495:errorcluster, "Device Details"=w492:T46, "Mercury Reference Out"=w496:T36)  [unwired: 1 in, 6 out]
        n191 = Unbundle By Name(w492) -> ("Manufacturing"=→"Manufacturing":T8, "Pressure Signals"=→"Pressure Signals":T11)
        n192 = call-poly <instrlib>:"Configuration (Read).vi"("error in"=w495, "Mercury Reference In"=w496) -> ("error out"=w500:errorcluster, "Nickname"=→"Nickname":string, "Mercury Reference Out"=w501:T36)  [unwired: 1 in, 6 out]
        n193 = call-poly <instrlib>:"Signals (Read).vi"("error in"=w500, "Mercury Reference In"=w501) -> ("error out"=w498:errorcluster, "Current"=→"Current":dbl, "Mercury Reference Out"=w499:T36)  [unwired: 1 in, 6 out]
        n194 = call-poly <instrlib>:"Signals (Read).vi"("error in"=w498, "Mercury Reference In"=w499) -> ("error out"=w491:errorcluster, "Voltage"=→"Voltage":dbl)  [unwired: 1 in, 7 out]
        n195 = call <vilib>:"Add State(s) to Queue__JKI_lib_State_Machine.vi"("State(s) in (\"\")"=w504) -> ("States Out"=w505:string)  [unwired: 14 in]
      }
      frame "Mercury: Query IPS: System" {
        # "Your code here.\n(You can make a copy of, or modify, this frame)"
        n196 = Unbundle By Name(w547) -> ("Mercury IPS Ref"=w508:T36)
        n197 = call-poly <instrlib>:"Configuration (Read).vi"("error in"=w513, "Mercury Reference In"=w508) -> ("error out"=w533:errorcluster, "Devices"=→"IPS Devices":string[], "Mercury Reference Out"=w532:T36)  [unwired: 1 in, 6 out]
        n198 = call-poly <instrlib>:"Configuration (Read).vi"("error in"=w533, "Mercury Reference In"=w532) -> ("error out"=w537:errorcluster, "Automatic Dimming"=→"Automatic Dimming 2":string, "Mercury Reference Out"=w536:T36)  [unwired: 1 in, 6 out]
        n199 = call-poly <instrlib>:"Configuration (Read).vi"("error in"=w537, "Mercury Reference In"=w536) -> ("error out"=w534:errorcluster, "Dimming Time"=→"Dimming Time 2":string, "Mercury Reference Out"=w535:T36)  [unwired: 1 in, 6 out]
        n200 = call-poly <instrlib>:"Configuration (Read).vi"("error in"=w534, "Mercury Reference In"=w535) -> ("error out"=w531:errorcluster, "Display Brightness"=→"Display Brightness 2":string, "Mercury Reference Out"=w530:T36)  [unwired: 1 in, 6 out]
        n201 = call-poly <instrlib>:"Configuration (Read).vi"("error in"=w531, "Mercury Reference In"=w530) -> ("error out"=w540:errorcluster, "Date"=→"Date 2":string, "Mercury Reference Out"=w541:T36)  [unwired: 1 in, 6 out]
        n202 = call-poly <instrlib>:"Configuration (Read).vi"("error in"=w540, "Mercury Reference In"=w541) -> ("error out"=w538:errorcluster, "Time"=→"Time 2":string, "Mercury Reference Out"=w539:T36)  [unwired: 1 in, 6 out]
        n203 = call-poly <instrlib>:"Configuration (Read).vi"("error in"=w538, "Mercury Reference In"=w539) -> ("error out"=w512:errorcluster, "time stamp"=→"time stamp 2":timestamp, "Mercury Reference Out"=w509:T36)  [unwired: 1 in, 6 out]
        n204 = call-poly <instrlib>:"Configuration (Read).vi"("error in"=w512, "Mercury Reference In"=w509) -> ("error out"=w514:errorcluster, "Hardware Version"=→"Hardware Version 2":string, "Mercury Reference Out"=w515:T36)  [unwired: 1 in, 6 out]
        n205 = call-poly <instrlib>:"Configuration (Read).vi"("error in"=w514, "Mercury Reference In"=w515) -> ("error out"=w516:errorcluster, "Firmware Version"=→"Firmware Version 2":string, "Mercury Reference Out"=w517:T36)  [unwired: 1 in, 6 out]
        n206 = call-poly <instrlib>:"Configuration (Read).vi"("error in"=w516, "Mercury Reference In"=w517) -> ("error out"=w522:errorcluster, "Serial Number"=→"Serial Number 2":string, "Mercury Reference Out"=w523:T36)  [unwired: 1 in, 6 out]
        n207 = call-poly <instrlib>:"Configuration (Read).vi"("error in"=w522, "Mercury Reference In"=w523) -> ("error out"=w518:errorcluster, "Free Space"=→"Free Space 2":i32, "Mercury Reference Out"=w519:T36)  [unwired: 1 in, 6 out]
        n208 = call-poly <instrlib>:"Configuration (Read).vi"("error in"=w518, "Mercury Reference In"=w519) -> ("error out"=w521:errorcluster, "Mode"=→"String 2":T32, "Mercury Reference Out"=w520:T36)  [unwired: 1 in, 6 out]
        n209 = Get Date/Time In Seconds() -> (seconds since 1Jan1904=w529:timestamp)
        n210 = call-poly <instrlib>:"Configuration (Set).vi"("error in"=w521, "time stamp"=w529, "Mercury Reference In"=w520) -> ("error out"=w511:errorcluster, "Response"=→"Set Date Response 2":T35)  [unwired: 1 in, 6 out]
        n211 = call <vilib>:"Add State(s) to Queue__JKI_lib_State_Machine.vi"("State(s) in (\"\")"=w549) -> ("States Out"=w548:string)  [unwired: 14 in]
      }
      frame "Mercury: Query IPS: LVL" {
        # "Level"
        n212 = Unbundle By Name(w589) -> ("Mercury IPS Ref"=w552:T36)
        n213 = local read "IPS Devices"() -> (w588:string[])
        n214 = Index Array(array=w588, index=0) -> (element=w551:string)
        n215 = call-poly <instrlib>:"Open.vi"("error in (no error)"=w558, "Device Identifier"=w551, "Mercury Reference In"=w552) -> ("error out"=w574:errorcluster, "Mercury Reference Out"=w573:T36)  [unwired: 7 out]
        n216 = call-poly <instrlib>:"Configuration (Read).vi"("error in"=w574, "Mercury Reference In"=w573) -> ("error out"=w579:errorcluster, "LVL Device Settings"=→"LVL Device DetailSettings":T14, "Mercury Reference Out"=w576:T36)  [unwired: 1 in, 6 out]
        n217 = call-poly <instrlib>:"Configuration (Read).vi"("error in"=w579, "Mercury Reference In"=w576) -> ("error out"=w580:errorcluster, "Serial Number"=→"LVL S/N":string, "Mercury Reference Out"=w578:T36)  [unwired: 1 in, 6 out]
        n218 = call-poly <instrlib>:"Configuration (Read).vi"("error in"=w580, "Mercury Reference In"=w578) -> ("error out"=w583:errorcluster, "Resistance Configuration"=→"He Res Config":T19, "Mercury Reference Out"=w582:T36)  [unwired: 1 in, 6 out]
        n219 = call-poly <instrlib>:"Configuration (Read).vi"("error in"=w583, "Mercury Reference In"=w582) -> ("error out"=w585:errorcluster, "Magnitude"=→"LVL P Magnitude":dbl, "Mercury Reference Out"=w584:T36)  [unwired: 1 in, 6 out]
        n220 = call-poly <instrlib>:"Configuration (Read).vi"("error in"=w585, "Mercury Reference In"=w584) -> ("error out"=w557:errorcluster, "Duration"=→"LVL P Duration":dbl, "Mercury Reference Out"=w555:T36)  [unwired: 1 in, 6 out]
        n221 = call-poly <instrlib>:"Configuration (Read).vi"("error in"=w557, "Mercury Reference In"=w555) -> ("error out"=w561:errorcluster, "Freq 100%"=→"N Freq 100%":dbl, "Mercury Reference Out"=w560:T36)  [unwired: 1 in, 6 out]
        n222 = call-poly <instrlib>:"Configuration (Read).vi"("error in"=w561, "Mercury Reference In"=w560) -> ("error out"=w564:errorcluster, "Pulse Period"=→"N Pulse Period":dbl, "Mercury Reference Out"=w563:T36)  [unwired: 1 in, 6 out]
        n223 = call-poly <instrlib>:"Signals (Read).vi"("error in"=w564, "Mercury Reference In"=w563) -> ("error out"=w566:errorcluster, "Resistance"=→"He Resistance":dbl, "Mercury Reference Out"=w565:T36)  [unwired: 1 in, 6 out]
        n224 = call-poly <instrlib>:"Signals (Read).vi"("error in"=w566, "Mercury Reference In"=w565) -> ("error out"=w568:errorcluster, "Level"=→"He Level" →"He LEVEL":dbl, "Mercury Reference Out"=w567:T36)  [unwired: 1 in, 6 out]
        n225 = call-poly <instrlib>:"Signals (Read).vi"("error in"=w568, "Mercury Reference In"=w567) -> ("error out"=w570:errorcluster, "Counter"=→"N Counter":u32, "Mercury Reference Out"=w569:T36)  [unwired: 1 in, 6 out]
        n226 = call-poly <instrlib>:"Signals (Read).vi"("error in"=w570, "Mercury Reference In"=w569) -> ("error out"=w556:errorcluster, "Level"=→"N Level" →"N2 LEVEL":dbl)  [unwired: 1 in, 7 out]
        n227 = call <vilib>:"Add State(s) to Queue__JKI_lib_State_Machine.vi"("State(s) in (\"\")"=w590) -> ("States Out"=w591:string)  [unwired: 14 in]
      }
      frame "Mercury: Query IPS: Temperature" {
        n228 = Unbundle By Name(w636) -> ("Mercury IPS Ref"=w597:T36)
        n229 = local read "IPS Devices"() -> (w635:string[])
        n230 = Index Array(array=w635, index=4) -> (element=w598:string)
        n231 = call-poly <instrlib>:"Open.vi"("error in (no error)"=w596, "Device Identifier"=w598, "Mercury Reference In"=w597) -> ("error out"=w623:errorcluster, "Mercury Reference Out"=w618:T36)  [unwired: 7 out]
        n232 = call-poly <instrlib>:"Configuration (Read).vi"("error in"=w623, "Mercury Reference In"=w618) -> ("error out"=w624:errorcluster, "Serial Number"=→"Temp S/N 2":string, "Mercury Reference Out"=w619:T36)  [unwired: 1 in, 6 out]
        n233 = call-poly <instrlib>:"Configuration (Read).vi"("error in"=w624, "Mercury Reference In"=w619) -> ("error out"=w625:errorcluster, "Nickname"=→"T Nickname 2":string, "Mercury Reference Out"=w620:T36)  [unwired: 1 in, 6 out]
        n234 = call-poly <instrlib>:"Configuration (Read).vi"("error in"=w625, "Mercury Reference In"=w620) -> ("error out"=w626:errorcluster, "Unit"=→"Unit 12":T3, "Excitation Magnitude"=→"Excitation Magnitude 2":dbl, "Mercury Reference Out"=w621:T36)  [unwired: 1 in, 5 out]
        n235 = call-poly <instrlib>:"Configuration (Read).vi"("error in"=w626, "Mercury Reference In"=w621) -> ("error out"=w627:errorcluster, "Sensor Type"=→"Sensor Type 2":T42, "Mercury Reference Out"=w622:T36)  [unwired: 1 in, 6 out]
        n236 = call-poly <instrlib>:"Configuration (Read).vi"("error in"=w627, "Mercury Reference In"=w622) -> ("error out"=w600:errorcluster, "Excitation Type"=→"Excitation Type 2":T7, "Mercury Reference Out"=w599:T36)  [unwired: 1 in, 6 out]
        n237 = call-poly <instrlib>:"Configuration (Read).vi"("error in"=w600, "Mercury Reference In"=w599) -> ("error out"=w605:errorcluster, "Unit"=→"H Unit 2":T3, "Hot Limit"=→"Hot Limit 2":dbl, "Mercury Reference Out"=w601:T36)  [unwired: 1 in, 5 out]
        n238 = call-poly <instrlib>:"Configuration (Read).vi"("error in"=w605, "Mercury Reference In"=w601) -> ("error out"=w606:errorcluster, "Unit"=→"C Unit 2":T3, "Cold Limit"=→"Cold Limit 2":dbl, "Mercury Reference Out"=w602:T36)  [unwired: 1 in, 5 out]
        n239 = call-poly <instrlib>:"Signals (Read).vi"("error in"=w606, "Mercury Reference In"=w602) -> ("error out"=w607:errorcluster, "Unit"=→"V Unit 2":T3, "Voltage"=→"Voltage 2":dbl, "Mercury Reference Out"=w603:T36)  [unwired: 1 in, 5 out]
        n240 = call-poly <instrlib>:"Signals (Read).vi"("error in"=w607, "Mercury Reference In"=w603) -> ("error out"=w608:errorcluster, "Unit"=→"T Unit 2":T3, "Temperature"=→"Temperature 2":dbl, "Mercury Reference Out"=w604:T36)  [unwired: 1 in, 5 out]
        n241 = call-poly <instrlib>:"Configuration (Read).vi"("error in"=w608, "Mercury Reference In"=w604) -> ("error out"=w609:errorcluster, "Device Details"=w592:T43)  [unwired: 1 in, 7 out]
        n242 = Unbundle By Name(w592) -> ("Manufacturing"=→"IPS Manufacturing":T8, "Excitation"=→"IPS Excitation":T6, "Calibration"=→"IPS Calibration":T4)
        n243 = call <vilib>:"Add State(s) to Queue__JKI_lib_State_Machine.vi"("State(s) in (\"\")"=w637) -> ("States Out"=w638:string)  [unwired: 14 in]
      }
      frame "Mercury: Query IPS: Magnet" {
        n244 = Unbundle By Name(w677) -> ("Mercury IPS Ref"=w643:T36)
        n245 = call-poly <instrlib>:"Open.vi"("error in (no error)"=w639, "Device Identifier"="Device Identifier", "Mercury Reference In"=w643) -> ("error out"=w662:errorcluster, "Mercury Reference Out"=w661:T36)  [unwired: 7 out]
        n246 = call-poly <instrlib>:"Configuration (Read).vi"("error in"=w662, "Mercury Reference In"=w661) -> ("error out"=w665:errorcluster, "Magnet Device Details"=→"Magnet Device Details":T22, "Mercury Reference Out"=w664:T36)  [unwired: 1 in, 6 out]
        n247 = call-poly <instrlib>:"Configuration (Read).vi"("error in"=w665, "Mercury Reference In"=w664) -> ("error out"=w668:errorcluster, "Serial Number"=→"Mag S/N":string, "Mercury Reference Out"=w667:T36)  [unwired: 1 in, 6 out]
        n248 = call-poly <instrlib>:"Configuration (Read).vi"("error in"=w668, "Mercury Reference In"=w667) -> ("error out"=w671:errorcluster, "Bipolar Output"=→"Bipolar Output":string, "Mercury Reference Out"=w670:T36)  [unwired: 1 in, 6 out]
        n249 = call-poly <instrlib>:"Configuration (Read).vi"("error in"=w671, "Mercury Reference In"=w670) -> ("error out"=w674:errorcluster, "Out Config"=→"Out Config":T51, "Mercury Reference Out"=w673:T36)  [unwired: 1 in, 6 out]
        n250 = call-poly <instrlib>:"Configuration (Read).vi"("error in"=w674, "Mercury Reference In"=w673) -> ("error out"=w645:errorcluster, "Unit"=→"Unit 8":T3, "Current Limit"=→"Current Limit":dbl, "Mercury Reference Out"=w642:T36)  [unwired: 1 in, 5 out]
        n251 = call-poly <instrlib>:"Configuration (Read).vi"("error in"=w645, "Mercury Reference In"=w642) -> ("error out"=w648:errorcluster, "Unit"=→"Unit 9":T3, "AtoB"=→"AtoB":dbl, "Mercury Reference Out"=w647:T36)  [unwired: 1 in, 5 out]
        n252 = call-poly <instrlib>:"Configuration (Read).vi"("error in"=w648, "Mercury Reference In"=w647) -> ("error out"=w651:errorcluster, "Switch Present"=→"Switch Present":string, "Mercury Reference Out"=w650:T36)  [unwired: 1 in, 6 out]
        n253 = call-poly <instrlib>:"Configuration (Read).vi"("error in"=w651, "Mercury Reference In"=w650) -> ("error out"=w656:errorcluster, "Unit"=→"Unit 10":T3, "SW VLIM"=→"SW VLIM":dbl, "Mercury Reference Out"=w655:T36)  [unwired: 1 in, 5 out]
        n254 = call-poly <instrlib>:"Signals (Read).vi"("error in"=w656, "Mercury Reference In"=w655) -> ("error out"=w658:errorcluster, "Unit"=→"Unit 11":T3, "Current Rate"=→"Current Rate":dbl, "Mercury Reference Out"=w657:T36)  [unwired: 1 in, 5 out]
        n255 = call-poly <instrlib>:"Signals (Read).vi"("error in"=w658, "Mercury Reference In"=w657) -> ("error out"=w644:errorcluster, "PSU Act Stat"=→"PSU Act Stat":T31)  [unwired: 1 in, 7 out]
        n256 = call <vilib>:"Add State(s) to Queue__JKI_lib_State_Machine.vi"("State(s) in (\"\")"=w678) -> ("States Out"=w679:string)  [unwired: 14 in]
      }
      frame "---------- Mercury: Idle ----------" {
        n257 = call <vilib>:"Add State(s) to Queue__JKI_lib_State_Machine.vi"("State(s) in (\"\")"=w683) -> ("States Out"=w682:string)  [unwired: 14 in]
      }
      frame "Mercury: Idle" {
        n258 = Unbundle By Name(w687) -> ("LEDs"=w685:bool[], "Mercury IPS Ref"=w704:T36, "Mercury ITC Ref"=w703:T36)
        n259 = Not(x=w685) -> (.not. x?=w684:bool[])
        "LEDs" <- w684
        n260 = disable-structure shown="Enabled" {
          disable-tunnel: w703 -> [w721 _]
          disable-tunnel: w702 -> [w720 w730]
          disable-tunnel: [w708 w730] -> w698
          frame Enabled {
            n261 = local read "ITC Devices"() -> (w718:string[])
            n262 = Index Array(array=w718, index=3) -> (element=w711:string)
            n263 = call-poly <instrlib>:"Open.vi"("error in (no error)"=w720, "Device Identifier"=w711, "Mercury Reference In"=w721) -> ("error out"=w717:errorcluster, "Mercury Reference Out"=w715:T36)  [unwired: 7 out]
            n264 = call-poly <instrlib>:"Signals (Read).vi"("error in"=w717, "Mercury Reference In"=w715) -> ("error out"=w714:errorcluster, "Temperature"=→"LPF Temperature":dbl, "Mercury Reference Out"=w713:T36)  [unwired: 1 in, 6 out]
            n265 = call-poly <instrlib>:"Signals (Read).vi"("error in"=w714, "Mercury Reference In"=w713) -> ("error out"=w710:errorcluster, "Resistance"=→"LPF Resistance":dbl, "Mercury Reference Out"=w709:T36)  [unwired: 1 in, 6 out]
            n266 = First Call?() -> (First Call?: T/F=w707:bool)
            n267 = case shown="False" w707 {
              tunnel: w710 -> [w722 w728]
              tunnel: w709 -> [_ w727]
              tunnel: [w722 w725] -> w708
              frame False {
              }
              frame True {
                n268 = call-poly <instrlib>:"Configuration (Set).vi"("error in"=w728, "Excitation Magnitude"=20.0, "Mercury Reference In"=w727) -> ("error out"=w725:errorcluster, "Response"=w724:T35)  [unwired: 5 in, 2 out]
                n269 = call "MercuryStateHistory.vi"("Current State in"=w724) -> ("delimited string"=w723:string)  [unwired: 9 in, 1 out]
                n270 = local write "Magnet Status 2"(w723) -> ()
              }
            }
          }
          frame Disabled {
            w729 = -1.0 ("LPF Temperature")
            n271 = local write "LPF Temperature"(w729) -> ()
            n272 = local write "LPF Resistance"(w729) -> ()
          }
        }
        n273 = local read "IPS Devices"() -> (w701:string[])
        n274 = Index Array(array=w701, index=5) -> (element=w699:string)
        n275 = Bundle By Name(cluster=w687, "LEDs"=w684) -> (w686:T39)
        n276 = call-poly <instrlib>:"Open.vi"("error in (no error)"=w698, "Device Identifier"=w699, "Mercury Reference In"=w704) -> ("error out"=w695:errorcluster, "Mercury Reference Out"=w696:T36)  [unwired: 7 out]
        n277 = call-poly <instrlib>:"Signals (Read).vi"("error in"=w695, "Mercury Reference In"=w696) -> ("error out"=w688:errorcluster, "Temperature"=→"Magnet Temperature":dbl, "Mercury Reference Out"=w697:T36)  [unwired: 1 in, 6 out]
        n278 = call-poly <instrlib>:"Signals (Read).vi"("error in"=w688, "Mercury Reference In"=w697) -> ("error out"=w691:errorcluster, "Resistance"=→"Magnet Resistance":dbl, "Mercury Reference Out"=w692:T36)  [unwired: 1 in, 6 out]
        n279 = First Call?() -> (First Call?: T/F=w689:bool)
        n280 = case shown="True" w689 {
          tunnel: [w731 w734] -> w690
          tunnel: w692 -> [_ w733]
          tunnel: w691 -> [w731 w732]
          frame False {
          }
          frame True {
            n281 = disable-structure shown="Disabled" {
              disable-tunnel: [w740 _] -> w734
              disable-tunnel: w733 -> [w736 _]
              disable-tunnel: w732 -> [w735 _]
              frame Disabled {
                n282 = call-poly <instrlib>:"Configuration (Set).vi"("error in"=w735, "Excitation Magnitude"=20.0, "Mercury Reference In"=w736) -> ("error out"=w740:errorcluster, "Response"=w738:T35)  [unwired: 5 in, 2 out]
                n283 = call "MercuryStateHistory.vi"("Current State in"=w738) -> ("delimited string"=w737:string)  [unwired: 9 in, 1 out]
                n284 = local write "Magnet Status 2"(w737) -> ()
              }
              frame Enabled {
              }
            }
          }
        }
        n285 = call <vilib>:"Add State(s) to Queue__JKI_lib_State_Machine.vi"("State(s) in (\"\")"=w705) -> ("States Out"=w706:string)  [unwired: 14 in]
      }
      frame "Mercury: IPS: Idle - 1" {
        # "set switch status"
        n286 = Unbundle By Name(w744) -> ("Mercury IPS Ref"=w747:T36)
        n287 = local read "Device Identifier"() -> (w760:T24)
        n288 = call-poly <instrlib>:"Configuration (Read).vi"("error in"=w775, "Mercury Reference In"=w747) -> ("error out"=w767:errorcluster, "Time"=w770:string, "Mercury Reference Out"=w768:T36)  [unwired: 1 in, 6 out]
        n289 = local write "Time 2"(w770) -> ()
        n290 = call-poly <instrlib>:"Open.vi"("error in (no error)"=w767, "Device Identifier"=w760, "Mercury Reference In"=w768) -> ("error out"=w766:errorcluster, "Mercury Reference Out"=w765:T36)  [unwired: 7 out]
        n291 = call-poly <instrlib>:"Signals (Read).vi"("error in"=w766, "Mercury Reference In"=w765) -> ("error out"=w742:errorcluster, "Switch Heater Status"=w746:string, "Mercury Reference Out"=w741:T36)  [unwired: 1 in, 6 out]
        n292 = Equal?(x=w746, y="ON") -> (x = y?=→"SWITCH HEATER":bool)
        n293 = call-poly <instrlib>:"Signals (Read).vi"("error in"=w742, "Mercury Reference In"=w741) -> ("error out"=w774:errorcluster, "Current"=→"Current (A)" →"Current (A)":dbl, "Mercury Reference Out"=w772:T36)  [unwired: 1 in, 6 out]
        n294 = call-poly <instrlib>:"Signals (Read).vi"("error in"=w774, "Mercury Reference In"=w772) -> ("error out"=w759:errorcluster, "Voltage"=→"Voltage (V)" →"Voltage (V)":dbl, "Mercury Reference Out"=w758:T36)  [unwired: 1 in, 6 out]
        n295 = call-poly <instrlib>:"Signals (Read).vi"("error in"=w759, "Mercury Reference In"=w758) -> ("error out"=w761:errorcluster, "Field"=→"Power Supply Field (T)":dbl, "Mercury Reference Out"=w764:T36)  [unwired: 1 in, 6 out]
        n296 = call-poly <instrlib>:"Signals (Read).vi"("error in"=w761, "Mercury Reference In"=w764) -> ("error out"=w762:errorcluster, "Target Field Rate"=→"Target Field Rate (T/min)":dbl, "Mercury Reference Out"=w763:T36)  [unwired: 1 in, 6 out]
        n297 = call-poly <instrlib>:"Signals (Read).vi"("error in"=w762, "Mercury Reference In"=w763) -> ("error out"=w757:errorcluster, "Target Field"=→"Target Field (T)":dbl, "Mercury Reference Out"=w756:T36)  [unwired: 1 in, 6 out]
        n298 = call-poly <instrlib>:"Signals (Read).vi"("error in"=w757, "Mercury Reference In"=w756) -> ("error out"=w773:errorcluster, "Persistant Field"=→"Magnet Field (T)" →"Magnet Field (T)":dbl, "Mercury Reference Out"=w771:T36)  [unwired: 1 in, 6 out]
        n299 = call-poly <instrlib>:"Signals (Read).vi"("error in"=w773, "Mercury Reference In"=w771) -> ("error out"=w745:errorcluster, "PSU Act Stat"=w748:T31)  [unwired: 1 in, 7 out]
        n300 = local write "PSU Act Stat"(w748) -> ()
        n301 = case shown="\"HOLD\"" w748 {
          selector: w748 -> [w778 _ _ _ _]
          tunnel: [w778 "Holding" "Ramping to Setpoint" "Ramping to Zero" "Clamped"] -> w755
          frame Default {
          }
          frame "HOLD" {
          }
          frame "RTOS" {
          }
          frame "RTOZ" {
          }
          frame "CLMP" {
          }
        }
        "Magnet Status" <- w755
        n302 = call <vilib>:"Add State(s) to Queue__JKI_lib_State_Machine.vi"("State(s) in (\"\")"=w776) -> ("States Out"=w777:string)  [unwired: 14 in]
      }
      frame "Mercury: IPS: Idle - 1a" {
        n303 = local read "IPS Devices"() -> (w808:string[])
        n304 = Unbundle By Name(w812) -> ("Mercury IPS Ref"=w811:T36)
        n305 = for {
          tunnel: w808 -> [w816] mode=indexing
          tunnel: [w815] -> w807 mode=indexing
          n306 = Match Pattern(string=w816, regular expression=":PSU") -> (before substring=w815:string)  [unwired: 1 in, 3 out]
        }
        n307 = Index Array(array=w807, index #1=6 ("index")) -> (element #1=w809:string, element #2=w805:string, element #3=w806:string)  [unwired: 2 in]
        n308 = call-poly <instrlib>:"Open.vi"("error in (no error)"=w810, "Device Identifier"=w809, "Mercury Reference In"=w811) -> ("error out"=w787:errorcluster, "Mercury Reference Out"=w791:T36)  [unwired: 7 out]
        n309 = call-poly <instrlib>:"Signals (Read).vi"("error in"=w787, "Mercury Reference In"=w791) -> ("error out"=w793:errorcluster, "Current"=→"M1 Current":dbl, "Mercury Reference Out"=w792:T36)  [unwired: 1 in, 6 out]
        n310 = call-poly <instrlib>:"Signals (Read).vi"("error in"=w793, "Mercury Reference In"=w792) -> ("error out"=w785:errorcluster, "Voltage"=→"M1 Voltage":dbl)  [unwired: 1 in, 7 out]
        n311 = call-poly <instrlib>:"Open.vi"("error in (no error)"=w785, "Device Identifier"=w805, "Mercury Reference In"=w811) -> ("error out"=w788:errorcluster, "Mercury Reference Out"=w790:T36)  [unwired: 7 out]
        n312 = call-poly <instrlib>:"Signals (Read).vi"("error in"=w788, "Mercury Reference In"=w790) -> ("error out"=w796:errorcluster, "Current"=→"M2 Current":dbl, "Mercury Reference Out"=w794:T36)  [unwired: 1 in, 6 out]
        n313 = call-poly <instrlib>:"Signals (Read).vi"("error in"=w796, "Mercury Reference In"=w794) -> ("error out"=w783:errorcluster, "Voltage"=→"M2 Voltage":dbl)  [unwired: 1 in, 7 out]
        n314 = call-poly <instrlib>:"Open.vi"("error in (no error)"=w783, "Device Identifier"=w806, "Mercury Reference In"=w811) -> ("error out"=w786:errorcluster, "Mercury Reference Out"=w789:T36)  [unwired: 7 out]
        n315 = call-poly <instrlib>:"Signals (Read).vi"("error in"=w786, "Mercury Reference In"=w789) -> ("error out"=w797:errorcluster, "Current"=→"M3 Current":dbl, "Mercury Reference Out"=w795:T36)  [unwired: 1 in, 6 out]
        n316 = call-poly <instrlib>:"Signals (Read).vi"("error in"=w797, "Mercury Reference In"=w795) -> ("error out"=w784:errorcluster, "Voltage"=→"M3 Voltage":dbl)  [unwired: 1 in, 7 out]
        n317 = call <vilib>:"Add State(s) to Queue__JKI_lib_State_Machine.vi"("State(s) in (\"\")"=w813) -> ("States Out"=w814:string)  [unwired: 14 in]
      }
      frame "Mercury: IPS: Idle - 2" {
        w820 = enum16{"write", "read"}."write" ("Function")
        # "set all of these things"
        n318 = Unbundle By Name(w828) -> ("Mercury IPS Ref"=w840:T36)
        n319 = local read "IPS Devices"() -> (w865:string[])
        n320 = Index Array(array=w865, index=0) -> (element=w864:string)
        n321 = call-poly <instrlib>:"Open.vi"("error in (no error)"=w861, "Device Identifier"=w864, "Mercury Reference In"=w840) -> ("error out"=w867:errorcluster, "Mercury Reference Out"=w868:T36)  [unwired: 7 out]
        n322 = call-poly <instrlib>:"Signals (Read).vi"("error in"=w867, "Mercury Reference In"=w868) -> ("error out"=w869:errorcluster, "Level"=w852:dbl, "Mercury Reference Out"=w870:T36)  [unwired: 1 in, 6 out]
        "He LVL Chart" <- w852
        n323 = Greater?(x=w852, y=20.0) -> (0:w859:bool)
        n324 = Greater?(x=w852, y=50.0) -> (0:w860:bool)
        n325 = call-poly <instrlib>:"Signals (Read).vi"("error in"=w869, "Mercury Reference In"=w870) -> ("error out"=w818:errorcluster, "Level"=w851:dbl)  [unwired: 1 in, 7 out]
        "N2 LVL Chart" <- w851
        n326 = case shown="True" w859 {
          tunnel: [w878 u32 6618880] -> w849
          tunnel: w860 -> [w879 _]
          frame False {
            n327 = case shown="False" w879 {
              tunnel: [u32 16711680 u32 16776704] -> w878
              frame False {
              }
              frame True {
              }
            }
          }
          frame True {
          }
        }
        n328 = local write "He LEVEL"(w852) -> ()
        n329 = property on="He LVL Chart" class="Slide (strict)"("Fill Color"=w849) -> ()  [unwired: 2 in, 2 out]
        n330 = property on="He LEVEL" class="DigNum (strict)"("NumText.TextColor"=w849) -> ()  [unwired: 2 in, 2 out]
        n331 = local write "N2 LEVEL"(w851) -> ()
        n332 = local read "Target Field Rate (T/min)"() -> (w845:dbl)
        n333 = local read "Power Supply Field (T)"() -> (w843:dbl)
        n334 = Greater?(x=w851, y=20.0) -> (0:w854:bool)
        n335 = Greater?(x=w851, y=50.0) -> (0:w853:bool)
        n336 = local read "Magnet Field (T)"() -> (w842:dbl)
        n337 = local read "Target Field (T)"() -> (w844:dbl)
        n338 = local read "Current (A)"() -> (w847:dbl)
        n339 = local read "Voltage (V)"() -> (w846:dbl)
        n340 = local read "SWITCH HEATER"() -> (w829:bool)
        n341 = local read "PSU Act Stat"() -> (w821:string)
        n342 = case shown="True" w854 {
          tunnel: [w873 u32 6618880] -> w850
          tunnel: w853 -> [w874 _]
          frame False {
            n343 = case shown="False" w874 {
              tunnel: [u32 16711680 u32 16776704] -> w873
              frame False {
              }
              frame True {
              }
            }
          }
          frame True {
          }
        }
        n344 = local read "Magnet Temperature"() -> (w838:dbl)
        n345 = property on="N2 LVL Chart" class="Slide (strict)"("Fill Color"=w850) -> ()  [unwired: 2 in, 2 out]
        n346 = property on="N2 LEVEL" class="DigNum (strict)"("NumText.TextColor"=w850) -> ()  [unwired: 2 in, 2 out]
        n347 = Bundle By Name(cluster=T29 {"Magnet Field"=0.0, "PS Field"=0.0, "Target Field"=0.0, "Target Field Rate"=0.0, "Voltage"=0.0, "Current"=0.0, "Switch"=FALSE, "Mercury State"=""} ("Status"), "Magnet Field"=w842, "PS Field"=w843, "Target Field"=w844, "Target Field Rate"=w845, "Voltage"=w846, "Current"=w847, "Switch"=w829, "Mercury State"=w821) -> (w826:T29)
        n348 = local read "Magnet Resistance"() -> (w839:dbl)
        n349 = Select(t="ON", s=w829, f="OFF") -> (s? t:f=w819:string)
        n350 = local read "M1 Current"() -> (w837:dbl)
        n351 = local read "M1 Voltage"() -> (w836:dbl)
        n352 = local read "M2 Current"() -> (w835:dbl)
        n353 = local read "M2 Voltage"() -> (w834:dbl)
        n354 = local read "M3 Current"() -> (w833:dbl)
        n355 = local read "M3 Voltage"() -> (w832:dbl)
        n356 = call <userlib>:"FGV_PSP - Mercury Status.vi"("error in"=w818, "Function"=w820, "Status"=w826) -> ("error out"=w825:errorcluster)  [unwired: 3 in, 1 out]
        n357 = Bundle(cluster=T30 {"Magnet Field"=0.0, "PS Field"=0.0, "Target Field"=0.0, "Target Field Rate"=0.0, "Voltage"=0.0, "Current"=0.0}, "Magnet Field"=w842, "PS Field"=w843, "Target Field"=w844, "Target Field Rate"=w845, "Voltage"=w846, "Current"=w847) -> (w848:T30)
        n358 = call <userlib>:"FGV_PSP - Mercury Action Status.vi"("error in"=w825, "Function"=w820, "Mercury Status"=w821) -> ("error out"=w824:errorcluster)  [unwired: 3 in, 1 out]
        n359 = Cluster To Array(cluster=w848) -> (array=w823:dbl[])
        n360 = Build Array(w837, w836, w835, w834, w833, w832) -> (w822:dbl[])
        n361 = Build Array (concatenate)(w823, w851, w852, w838, w839, w822) -> (w863:dbl[])
        n362 = Build Array(w821, w819) -> (w862:string[])
        n363 = call "1820_IPS_to_DSC.vi"("str"=w862, "dbl"=w863) -> ()  [unwired: 2 in]
        n364 = call <vilib>:"Add State(s) to Queue__JKI_lib_State_Machine.vi"("State(s) in (\"\")"=w871) -> ("States Out"=w872:string)  [unwired: 14 in]
      }
      frame "Mercury: IPS: Idle - 3" {
        n365 = case shown="False" "Enable RS232 Panel" {
          tunnel: w885 -> [w889 w891]
          tunnel: [w889 w890] -> w884
          frame False {
          }
          frame True {
            n366 = call "Oxford_MNK_Omega_Sign.vi"("error in (no error)"=w891) -> ("error out"=w890:errorcluster)  [unwired: 10 in]
          }
        }
        n367 = call <vilib>:"Add State(s) to Queue__JKI_lib_State_Machine.vi"("State(s) in (\"\")"=w887) -> ("States Out"=w888:string)  [unwired: 14 in]
      }
      frame "Mercury: ITC: Idle" {
        n368 = Unbundle By Name(w913) -> ("Mercury ITC Ref"=w897:T36)
        n369 = local read "ITC Devices"() -> (w912:string[])
        n370 = Index Array(array=w912, index=1) -> (element=w910:string)
        n371 = call-poly <instrlib>:"Open.vi"("error in (no error)"=w892, "Device Identifier"=w910, "Mercury Reference In"=w897) -> ("error out"=w909:errorcluster, "Mercury Reference Out"=w908:T36)  [unwired: 7 out]
        n372 = call-poly <instrlib>:"Configuration (Read).vi"("error in"=w909, "Mercury Reference In"=w908) -> ("error out"=w906:errorcluster, "Device Details"=w907:T46)  [unwired: 1 in, 7 out]
        n373 = local read "ITC Devices"() -> (w904:string[])
        n374 = Unbundle By Name(w907) -> ("Pressure Signals.Pressure"=w896:string)
        n375 = Index Array(array=w904, index=0) -> (element=w903:string)
        n376 = Fract/Exp String To Number(string=w896) -> (number=w895:dbl)  [unwired: 3 in, 1 out]
        "LPF Pressure" <- w895
        n377 = call-poly <instrlib>:"Open.vi"("error in (no error)"=w906, "Device Identifier"=w903, "Mercury Reference In"=w897) -> ("error out"=w902:errorcluster, "Mercury Reference Out"=w901:T36)  [unwired: 7 out]
        n378 = local read "LPF Temperature"() -> (w894:dbl)
        n379 = local read "LPF Resistance"() -> (w893:dbl)
        n380 = call-poly <instrlib>:"Signals (Read).vi"("error in"=w902, "Mercury Reference In"=w901) -> ("error out"=w898:errorcluster, "% Open"=w899:dbl)  [unwired: 1 in, 7 out]
        "LPF Needle Valve (%)" <- w899
        n381 = Build Array(w894, w895, w899, w893) -> (w900:dbl[])
        n382 = call "1820_ITC_to_DSC.vi"("dbl"=w900) -> ()  [unwired: 3 in]
        n383 = call <vilib>:"Add State(s) to Queue__JKI_lib_State_Machine.vi"("State(s) in (\"\")"=w914) -> ("States Out"=w915:string)  [unwired: 14 in]
      }
      frame "Mercury: Empty" {
        n384 = call <vilib>:"Add State(s) to Queue__JKI_lib_State_Machine.vi"("State(s) in (\"\")"=w918) -> ("States Out"=w919:string)  [unwired: 14 in]
      }
      frame "---------- Mercury: Action ----------" {
        n385 = call <vilib>:"Add State(s) to Queue__JKI_lib_State_Machine.vi"("State(s) in (\"\")"=w923) -> ("States Out"=w922:string)  [unwired: 14 in]
      }
      frame "Mercury: Remote" {
        w939 = "\n"
        w932 = enum16{"write", "read"}."read" ("Function")
        n386 = call <userlib>:"FGV_PSP - Mercury Actions.vi"("error in"=w924, "Function"=w932) -> ("error out"=w937:errorcluster, "Actions"=w938:T52)  [unwired: 4 in]
        n387 = call <userlib>:"FGV_PSP - Mercury Targets.vi"("error in"=w937, "Function"=w932) -> ("error out"=w933:errorcluster, "Targets"=w936:T53)  [unwired: 4 in]
        n388 = Unbundle By Name(w936) -> ("Target Field (T)"=w935:dbl, "Target Field Rate (T/min)"=w934:dbl)
        n389 = Unbundle By Name(w938) -> ("Hold"=w931:bool, "Clamp"=w926:bool, "To Set"=w927:bool, "To Zero"=w928:bool, "PS Heat"=w929:bool, "Lambda"=w925:bool, "Send to IPS"=w930:bool)
        n390 = local read "Send to IPS"() -> (w953:bool)
        n391 = local read "Lambda"() -> (w952:bool)
        n392 = local read "To Zero"() -> (w950:bool)
        n393 = local read "PS Heat"() -> (w951:bool)
        n394 = local read "Clamp"() -> (w948:bool)
        n395 = local read "To Set"() -> (w949:bool)
        n396 = local read "Hold"() -> (w947:bool)
        n397 = local write "Send to IPS"(w930) -> ()
        n398 = local write "Lambda"(w925) -> ()
        n399 = local write "To Zero"(w928) -> ()
        n400 = local write "PS Heat"(w929) -> ()
        n401 = local write "Clamp"(w926) -> ()
        n402 = Not Equal?(x=w947, y=w931) -> (x != y?=w960:bool)
        n403 = Not Equal?(x=w948, y=w926) -> (x != y?=w959:bool)
        n404 = Not Equal?(x=w949, y=w927) -> (x != y?=w958:bool)
        n405 = local write "To Set"(w927) -> ()
        n406 = Not Equal?(x=w950, y=w928) -> (x != y?=w957:bool)
        n407 = Not Equal?(x=w951, y=w929) -> (x != y?=w956:bool)
        n408 = Not Equal?(x=w952, y=w925) -> (x != y?=w955:bool)
        n409 = Not Equal?(x=w953, y=w930) -> (x != y?=w954:bool)
        n410 = local write "Hold"(w931) -> ()
        n411 = local write "Target Field (T)"(w935) -> ()
        n412 = local write "Target Rate (T/min)"(w934) -> ()
        n413 = case shown="True" w960 {
          tunnel: ["" ("State(s) in Front (\"\")") "Mercury: Hold" ("State(s) in Front (\"\")")] -> w946
          frame False {
          }
          frame True {
          }
        }
        n414 = case shown="True" w958 {
          tunnel: ["" ("State(s) in Front (\"\")") "Mercury: To Set" ("State(s) in Front (\"\")")] -> w944
          frame False {
          }
          frame True {
          }
        }
        n415 = case shown="True" w956 {
          tunnel: ["" ("State(s) in Front (\"\")") "Mercury: PS Heat" ("State(s) in Front (\"\")")] -> w942
          frame False {
          }
          frame True {
          }
        }
        n416 = case shown="True" w955 {
          tunnel: ["" ("State(s) in Front (\"\")") "Mercury: Lambda" ("State(s) in Front (\"\")")] -> w941
          frame False {
          }
          frame True {
          }
        }
        n417 = case shown="True" w954 {
          tunnel: ["" ("State(s) in Front (\"\")") "Mercury: Send To IPS" ("State(s) in Front (\"\")")] -> w940
          frame False {
          }
          frame True {
          }
        }
        n418 = case shown="True" w959 {
          tunnel: ["" ("State(s) in Front (\"\")") "Mercury: Clamp" ("State(s) in Front (\"\")")] -> w945
          frame False {
          }
          frame True {
          }
        }
        n419 = case shown="True" w957 {
          tunnel: ["" ("State(s) in Front (\"\")") "Mercury: To Zero" ("State(s) in Front (\"\")")] -> w943
          frame False {
          }
          frame True {
          }
        }
        n420 = Concatenate Strings(w946, w939, w945, w939, w944, w939, w943, w939, w942, w939, w941, w939, w940, w939) -> (w962:string)
        n421 = call <vilib>:"Add State(s) to Queue__JKI_lib_State_Machine.vi"("State(s) in Front (\"\")"=w962, "State(s) in (\"\")"=w963) -> ("States Out"=w964:string)  [unwired: 13 in]
      }
      frame "Mercury: Hold" {
        w984 = FALSE ("Hold")
        n422 = Unbundle By Name(w987) -> ("Mercury IPS Ref"=w995:T36)
        n423 = local read "Device Identifier"() -> (w996:T24)
        n424 = call-poly <instrlib>:"Open.vi"("error in (no error)"=w993, "Device Identifier"=w996, "Mercury Reference In"=w995) -> ("error out"=w997:errorcluster, "Mercury Reference Out"=w994:T36)  [unwired: 7 out]
        n425 = call-poly <instrlib>:"Signals (Set).vi"("error in"=w997, "PSU Act Stat"=T31 "HOLD", "Mercury Reference In"=w994) -> ("error out"=w990:errorcluster, "Response"=w988:T35)  [unwired: 1 in, 6 out]
        n426 = call "IPSReplytoDSC.vi"("error in (no error)"=w990, "Response"=w988) -> ("error out"=w982:errorcluster)  [unwired: 9 in]
        n427 = call "MercuryStateHistory.vi"("initialize?"=FALSE, "Current State in"=w988) -> ("delimited string"=w991:string)  [unwired: 8 in, 1 out]
        n428 = local write "Magnet Status 2"(w991) -> ()
        n429 = local write "Hold"(w984) -> ()
        n430 = call <userlib>:"FGV_PSP - Mercury Actions.vi"("error in"=w982, "Function"=enum16{"write", "read"}."read") -> ("error out"=w981:errorcluster, "Actions"=w979:T52)  [unwired: 4 in]
        n431 = Bundle By Name(cluster=w979, "Hold"=w984) -> (w986:T52)
        n432 = call <userlib>:"FGV_PSP - Mercury Actions.vi"("error in"=w981, "Function"=enum16{"write", "read"}."write", "Actions"=w986) -> ("error out"=w983:errorcluster)  [unwired: 3 in, 1 out]
        n433 = call <vilib>:"Add State(s) to Queue__JKI_lib_State_Machine.vi"("State(s) in (\"\")"=w998) -> ("States Out"=w999:string)  [unwired: 14 in]
      }
      frame "Mercury: Heater Current" {
        n434 = Unbundle By Name(w1025) -> ("Mercury IPS Ref"=w1028:T36)
        n435 = local read "Device Identifier"() -> (w1029:T24)
        n436 = call-poly <instrlib>:"Open.vi"("error in (no error)"=w1022, "Device Identifier"=w1029, "Mercury Reference In"=w1028) -> ("Mercury Reference Out"=w1021:T36)  [unwired: 8 out]
        n437 = call-poly <instrlib>:"Configuration (Set).vi"("error in"=w1022, "Password"="abc123", "Mode"=T32 "ENG", "Mercury Reference In"=w1021) -> ("error out"=w1019:errorcluster, "Response"=w1020:T35, "Mercury Reference Out"=w1017:T36)  [unwired: 4 in, 1 out]
        n438 = call "IPSReplytoDSC.vi"("error in (no error)"=w1019, "Response"=w1020) -> ("error out"=w1015:errorcluster)  [unwired: 9 in]
        n439 = call "MercuryStateHistory.vi"("initialize?"=FALSE, "Current State in"=w1020) -> ("delimited string"=w1027:string)  [unwired: 8 in, 1 out]
        n440 = local write "Magnet Status 2"(w1027) -> ()
        n441 = call <userlib>:"Wait (ms)__ogtk.vi"("error in (no error)"=w1015, "milliseconds to wait"=u32 1000) -> ("error out"=w1016:errorcluster)  [unwired: 8 in, 1 out]
        n442 = call-poly <instrlib>:"Configuration (Set).vi"("error in"=w1016, "Swh Htr Current"="Swh Htr Current (mA)", "Mercury Reference In"=w1017) -> ("error out"=w1011:errorcluster, "Response"=w1001:T35, "Mercury Reference Out"=w1006:T36)  [unwired: 5 in, 1 out]
        n443 = call "IPSReplytoDSC.vi"("error in (no error)"=w1011, "Response"=w1001) -> ("error out"=w1010:errorcluster)  [unwired: 9 in]
        n444 = call "MercuryStateHistory.vi"("initialize?"=FALSE, "Current State in"=w1001) -> ("delimited string"=w1004:string)  [unwired: 8 in, 1 out]
        n445 = local write "Magnet Status 2"(w1004) -> ()
        n446 = call <userlib>:"Wait (ms)__ogtk.vi"("error in (no error)"=w1010, "milliseconds to wait"=u32 1000) -> ("error out"=w1009:errorcluster)  [unwired: 8 in, 1 out]
        n447 = call-poly <instrlib>:"Configuration (Set).vi"("error in"=w1009, "Mode"=T32 "NORM", "Mercury Reference In"=w1006) -> ("error out"=w1008:errorcluster, "Response"=w1000:T35)  [unwired: 5 in, 2 out]
        n448 = call "IPSReplytoDSC.vi"("error in (no error)"=w1008, "Response"=w1000) -> ("error out"=w1007:errorcluster)  [unwired: 9 in]
        n449 = call "MercuryStateHistory.vi"("initialize?"=FALSE, "Current State in"=w1000) -> ("delimited string"=w1003:string)  [unwired: 8 in, 1 out]
        n450 = local write "Magnet Status 2"(w1003) -> ()
        n451 = call <vilib>:"Add State(s) to Queue__JKI_lib_State_Machine.vi"("State(s) in (\"\")"=w1030) -> ("States Out"=w1031:string)  [unwired: 14 in]
      }
      frame "Mercury: Clamp" {
        w1036 = FALSE
        n452 = Unbundle By Name(w1040) -> ("Mercury IPS Ref"=w1047:T36)
        n453 = local read "Device Identifier"() -> (w1050:T24)
        n454 = call-poly <instrlib>:"Open.vi"("error in (no error)"=w1046, "Device Identifier"=w1050, "Mercury Reference In"=w1047) -> ("error out"=w1049:errorcluster, "Mercury Reference Out"=w1048:T36)  [unwired: 7 out]
        n455 = call-poly <instrlib>:"Signals (Set).vi"("error in"=w1049, "PSU Act Stat"=T31 "CLMP", "Mercury Reference In"=w1048) -> ("error out"=w1044:errorcluster, "Response"=w1041:T35)  [unwired: 1 in, 6 out]
        n456 = call "IPSReplytoDSC.vi"("error in (no error)"=w1044, "Response"=w1041) -> ("error out"=w1035:errorcluster)  [unwired: 9 in]
        n457 = call "MercuryStateHistory.vi"("initialize?"=FALSE, "Current State in"=w1041) -> ("delimited string"=w1042:string)  [unwired: 8 in, 1 out]
        n458 = local write "Magnet Status 2"(w1042) -> ()
        n459 = local write "Clamp"(w1036) -> ()
        n460 = call <userlib>:"FGV_PSP - Mercury Actions.vi"("error in"=w1035, "Function"=enum16{"write", "read"}."read") -> ("error out"=w1033:errorcluster, "Actions"=w1032:T52)  [unwired: 4 in]
        n461 = Bundle By Name(cluster=w1032, "Clamp"=w1036) -> (w1039:T52)
        n462 = call <userlib>:"FGV_PSP - Mercury Actions.vi"("error in"=w1033, "Function"=enum16{"write", "read"}."write", "Actions"=w1039) -> ("error out"=w1037:errorcluster)  [unwired: 3 in, 1 out]
        n463 = call <vilib>:"Add State(s) to Queue__JKI_lib_State_Machine.vi"("State(s) in (\"\")"=w1051) -> ("States Out"=w1052:string)  [unwired: 14 in]
      }
      frame "Mercury: To Set" {
        w1059 = FALSE
        n464 = Unbundle By Name(w1061) -> ("Mercury IPS Ref"=w1069:T36)
        n465 = local read "Device Identifier"() -> (w1068:T24)
        n466 = call-poly <instrlib>:"Open.vi"("error in (no error)"=w1067, "Device Identifier"=w1068, "Mercury Reference In"=w1069) -> ("error out"=w1070:errorcluster, "Mercury Reference Out"=w1071:T36)  [unwired: 7 out]
        n467 = call-poly <instrlib>:"Signals (Set).vi"("error in"=w1070, "PSU Act Stat"=T31 "RTOS", "Mercury Reference In"=w1071) -> ("error out"=w1064:errorcluster, "Response"=w1063:T35)  [unwired: 1 in, 6 out]
        n468 = call "IPSReplytoDSC.vi"("error in (no error)"=w1064, "Response"=w1063) -> ("error out"=w1055:errorcluster)  [unwired: 9 in]
        n469 = call "MercuryStateHistory.vi"("initialize?"=FALSE, "Current State in"=w1063) -> ("delimited string"=w1065:string)  [unwired: 8 in, 1 out]
        n470 = local write "Magnet Status 2"(w1065) -> ()
        n471 = call <userlib>:"FGV_PSP - Mercury Actions.vi"("error in"=w1055, "Function"=enum16{"write", "read"}."read") -> ("error out"=w1054:errorcluster, "Actions"=w1053:T52)  [unwired: 4 in]
        n472 = local write "To Set"(w1059) -> ()
        n473 = Bundle By Name(cluster=w1053, "To Set"=w1059) -> (w1060:T52)
        n474 = call <userlib>:"FGV_PSP - Mercury Actions.vi"("error in"=w1054, "Function"=enum16{"write", "read"}."write", "Actions"=w1060) -> ("error out"=w1058:errorcluster)  [unwired: 3 in, 1 out]
        n475 = call <vilib>:"Add State(s) to Queue__JKI_lib_State_Machine.vi"("State(s) in (\"\")"=w1072) -> ("States Out"=w1073:string)  [unwired: 14 in]
      }
      frame "Mercury: To Zero" {
        w1080 = FALSE
        n476 = Unbundle By Name(w1082) -> ("Mercury IPS Ref"=w1090:T36)
        n477 = local read "Device Identifier"() -> (w1089:T24)
        n478 = call-poly <instrlib>:"Open.vi"("error in (no error)"=w1088, "Device Identifier"=w1089, "Mercury Reference In"=w1090) -> ("error out"=w1091:errorcluster, "Mercury Reference Out"=w1092:T36)  [unwired: 7 out]
        n479 = call-poly <instrlib>:"Signals (Set).vi"("error in"=w1091, "PSU Act Stat"=T31 "RTOZ", "Mercury Reference In"=w1092) -> ("error out"=w1085:errorcluster, "Response"=w1083:T35)  [unwired: 1 in, 6 out]
        n480 = call "IPSReplytoDSC.vi"("error in (no error)"=w1085, "Response"=w1083) -> ("error out"=w1078:errorcluster)  [unwired: 9 in]
        n481 = call "MercuryStateHistory.vi"("initialize?"=FALSE, "Current State in"=w1083) -> ("delimited string"=w1086:string)  [unwired: 8 in, 1 out]
        n482 = local write "Magnet Status 2"(w1086) -> ()
        n483 = local write "To Zero"(w1080) -> ()
        n484 = call <userlib>:"FGV_PSP - Mercury Actions.vi"("error in"=w1078, "Function"=enum16{"write", "read"}."read") -> ("error out"=w1077:errorcluster, "Actions"=w1076:T52)  [unwired: 4 in]
        n485 = Bundle By Name(cluster=w1076, "To Zero"=w1080) -> (w1081:T52)
        n486 = call <userlib>:"FGV_PSP - Mercury Actions.vi"("error in"=w1077, "Function"=enum16{"write", "read"}."write", "Actions"=w1081) -> ("error out"=w1079:errorcluster)  [unwired: 3 in, 1 out]
        n487 = call <vilib>:"Add State(s) to Queue__JKI_lib_State_Machine.vi"("State(s) in (\"\")"=w1093) -> ("States Out"=w1094:string)  [unwired: 14 in]
      }
      frame "Mercury: PS Heat" {
        # "set switch action to F because we\nalready changed it"
        # "set the status of the switch\nT = ON\nF = OFF"
        n488 = local read "Device Identifier"() -> (w1106:T24)
        n489 = Unbundle By Name(w1101) -> ("Mercury IPS Ref"=w1107:T36)
        n490 = call-poly <instrlib>:"Open.vi"("error in (no error)"=w1103, "Device Identifier"=w1106, "Mercury Reference In"=w1107) -> ("error out"=w1104:errorcluster, "Mercury Reference Out"=w1105:T36)  [unwired: 7 out]
        n491 = call-poly <instrlib>:"Signals (Read).vi"("error in"=w1104, "Mercury Reference In"=w1105) -> ("error out"=w1109:errorcluster, "Current"=w1098:dbl, "Mercury Reference Out"=w1108:T36)  [unwired: 1 in, 6 out]
        n492 = call-poly <instrlib>:"Signals (Read).vi"("error in"=w1109, "Mercury Reference In"=w1108) -> ("error out"=w1110:errorcluster, "Persistant Current"=w1097:dbl, "Mercury Reference Out"=w1095:T36)  [unwired: 1 in, 6 out]
        n493 = Subtract(x=w1097, y=w1098) -> (x-y=w1111:dbl)
        n494 = Absolute Value(x=w1111) -> (abs(x)=w1112:dbl)
        n495 = Less?(x=w1112, y=0.1) -> (x < y?=w1114:bool)
        n496 = case shown="False" w1114 {
          selector: w1114 -> [_ w1119]
          tunnel: [w1118 w1119] -> w1096
          frame False {
            n497 = Two Button Dialog(message="The magnet current is more\nthan 0.1A different to the\nPSU output current.  It is not\nadvisable to switch on the\nswitch heater unless these\ncurrents are equal!") -> (T button?=w1118:bool)  [unwired: 2 out]
          }
          frame True {
          }
        }
        n498 = local read "PS Heat"() -> (w1100:bool)
        n499 = Or(x=w1096, y=w1100) -> (x .or. y?=w1099:bool)
        n500 = case shown="True" w1099 {
          tunnel: w1095 -> [_ w1151]
          tunnel: w1110 -> [w1120 w1150]
          tunnel: [w1120 w1139] -> w1102
          frame False {
          }
          frame True {
            w1124 = FALSE ("PS Heat")
            n501 = Get Date/Time In Seconds() -> (seconds since 1Jan1904=→"PS ON/OFF":timestamp)
            n502 = call-poly <instrlib>:"Signals (Read).vi"("error in"=w1150, "Mercury Reference In"=w1151) -> ("error out"=w1152:errorcluster, "Switch Heater Status"=w1136:string, "Mercury Reference Out"=w1137:T36)  [unwired: 1 in, 6 out]
            n503 = Equal?(x=w1136, y="ON") -> (x = y?=w1134:bool)
            n504 = call <userlib>:"Wait (ms)__ogtk.vi"("error in (no error)"=w1152, "milliseconds to wait"=u32 100 ("millisecond multiple")) -> ("error out"=w1149:errorcluster)  [unwired: 8 in, 1 out]
            n505 = Select(t=T33 "OFF" ("Set Switch Heater"), s=w1134, f=T33 "ON" ("Set Switch Heater")) -> (s? t:f=w1129:T33)
            n506 = call-poly <instrlib>:"Signals (Set).vi"("error in"=w1149, "Set Switch Heater"=w1129, "Mercury Reference In"=w1137) -> ("error out"=w1143:errorcluster, "Response"=w1141:T35, "Mercury Reference Out"=w1133:T36)  [unwired: 1 in, 5 out]
            n507 = call "MercuryStateHistory.vi"("initialize?"=FALSE, "Current State in"=w1141) -> ("delimited string"=w1145:string)  [unwired: 8 in, 1 out]
            n508 = local write "Magnet Status 2"(w1145) -> ()
            n509 = call "IPSReplytoDSC.vi"("error in (no error)"=w1143, "Response"=w1141) -> ("error out"=w1140:errorcluster)  [unwired: 9 in]
            n510 = while {
              tunnel: [w1160] -> w1138
              tunnel: w1140 -> [w1158]
              tunnel: w1129 -> [w1156]
              tunnel: w1133 -> [w1154]
              tunnel: [w1153] -> w1128
              stop <- w1155 stop-if-true
              # "wait here while setting"
              n511 = call-poly <instrlib>:"Signals (Read).vi"("error in"=w1158, "Mercury Reference In"=w1154) -> ("error out"=w1160:errorcluster, "Switch Heater Status"=w1157:string)  [unwired: 1 in, 7 out]
              n512 = Equal?(x=w1157, y=w1156) -> (x = y?=w1155:bool)
              n513 = Equal?(x=w1157, y="ON") -> (x = y?=w1153:bool)
            }
            n514 = Bundle By Name(cluster=T29 {"Magnet Field"=0.0, "PS Field"=0.0, "Target Field"=0.0, "Target Field Rate"=0.0, "Voltage"=0.0, "Current"=0.0, "Switch"=FALSE, "Mercury State"=""} ("Status"), "Switch"=w1128) -> (w1131:T29)
            n515 = call <userlib>:"FGV_PSP - Mercury Status.vi"("error in"=w1138, "Function"=enum16{"write", "read"}."write", "Status"=w1131) -> ("error out"=w1126:errorcluster)  [unwired: 3 in, 1 out]
            n516 = local write "PS Heat"(w1124) -> ()
            n517 = call <userlib>:"FGV_PSP - Mercury Actions.vi"("error in"=w1126, "Function"=enum16{"write", "read"}."read") -> ("error out"=w1125:errorcluster, "Actions"=w1123:T52)  [unwired: 4 in]
            n518 = Bundle By Name(cluster=w1123, "PS Heat"=w1124) -> (w1122:T52)
            n519 = call <userlib>:"FGV_PSP - Mercury Actions.vi"("error in"=w1125, "Function"=enum16{"write", "read"}."write", "Actions"=w1122) -> ("error out"=w1139:errorcluster)  [unwired: 3 in, 1 out]
          }
        }
        n520 = call <vilib>:"Add State(s) to Queue__JKI_lib_State_Machine.vi"("State(s) in (\"\")"=w1115) -> ("States Out"=w1116:string)  [unwired: 14 in]
      }
      frame "Mercury: Send To IPS" {
        w1167 = FALSE
        n521 = local read "Device Identifier"() -> (w1185:T24)
        n522 = Unbundle By Name(w1172) -> ("Mercury IPS Ref"=w1184:T36)
        n523 = call-poly <instrlib>:"Open.vi"("error in (no error)"=w1182, "Device Identifier"=w1185, "Mercury Reference In"=w1184) -> ("error out"=w1186:errorcluster, "Mercury Reference Out"=w1183:T36)  [unwired: 7 out]
        n524 = call-poly <instrlib>:"Signals (Set).vi"("error in"=w1186, "Target Field Rate"="Target Rate (T/min)", "Mercury Reference In"=w1183) -> ("error out"=w1180:errorcluster, "Response"=w1178:T35, "Mercury Reference Out"=w1171:T36)  [unwired: 2 in, 4 out]
        n525 = call "MercuryStateHistory.vi"("initialize?"=FALSE, "Current State in"=w1178) -> ("delimited string"=w1174:string)  [unwired: 8 in, 1 out]
        n526 = call "IPSReplytoDSC.vi"("error in (no error)"=w1180, "Response"=w1178) -> ("error out"=w1179:errorcluster)  [unwired: 9 in]
        n527 = local write "Magnet Status 2"(w1174) -> ()
        n528 = call-poly <instrlib>:"Signals (Set).vi"("error in"=w1179, "Target Field"="Target Field (T)", "Mercury Reference In"=w1171) -> ("error out"=w1181:errorcluster, "Response"=w1173:T35)  [unwired: 2 in, 5 out]
        n529 = call "IPSReplytoDSC.vi"("error in (no error)"=w1181, "Response"=w1173) -> ("error out"=w1163:errorcluster)  [unwired: 9 in]
        n530 = call "MercuryStateHistory.vi"("initialize?"=FALSE, "Current State in"=w1173) -> ("delimited string"=w1175:string)  [unwired: 8 in, 1 out]
        n531 = local write "Magnet Status 2"(w1175) -> ()
        n532 = call <userlib>:"FGV_PSP - Mercury Actions.vi"("error in"=w1163, "Function"=enum16{"write", "read"}."read") -> ("error out"=w1162:errorcluster, "Actions"=w1161:T52)  [unwired: 4 in]
        n533 = local write "Send to IPS"(w1167) -> ()
        n534 = Bundle By Name(cluster=w1161, "Send to IPS"=w1167) -> (w1168:T52)
        n535 = call <userlib>:"FGV_PSP - Mercury Actions.vi"("error in"=w1162, "Function"=enum16{"write", "read"}."write", "Actions"=w1168) -> ("error out"=w1166:errorcluster)  [unwired: 3 in, 1 out]
        n536 = call <vilib>:"Add State(s) to Queue__JKI_lib_State_Machine.vi"("State(s) in (\"\")"=w1187) -> ("States Out"=w1188:string)  [unwired: 14 in]
      }
      frame "Mercury: Lambda" {
        # "AUX\nPRES\nHTR\nTEMP"
        n537 = Unbundle By Name(w1197) -> ("Mercury ITC Ref"=w1209:T36)
        n538 = local read "Lambda"() -> (w1195:bool)
        n539 = call-poly <instrlib>:"Open.vi"("error in (no error)"=w1198, "Device Identifier"="lambda:LPC", "Mercury Reference In"=w1209) -> ("error out"=w1206:errorcluster, "Mercury Reference Out"=w1205:T36)  [unwired: 7 out]
        n540 = Select(t="ON" ("Sweep Mode"), s=w1195, f="OFF" ("Sweep Mode")) -> (s? t:f=w1204:string)
        n541 = case shown="False" w1195 {
          frame False {
            n542 = disable-structure shown="Disabled" {
              frame Disabled {
                n543 = property on="Close Needle Valve" class="Bool (strict)"("Val(Sgnl)"=TRUE ("Value (Signaling)")) -> ()  [unwired: 2 in, 2 out]
              }
              frame Enabled {
              }
            }
          }
          frame True {
          }
        }
        n544 = case shown="False" w1195 {
          frame False {
            n545 = local write "LPF ON"(timestamp(0 s since 1904-01-01) ("LPF ON")) -> ()
          }
          frame True {
            n546 = Get Date/Time In Seconds() -> (seconds since 1Jan1904=w1214:timestamp)
            n547 = local write "LPF ON"(w1214) -> ()
          }
        }
        n548 = call-poly <instrlib>:"Configuration (Set).vi"("error in"=w1206, "Lambda Auto"=w1204, "Mercury Reference In"=w1205) -> ("error out"=w1202:errorcluster, "Response"=w1201:T35)  [unwired: 5 in, 2 out]
        n549 = call "ITCReplytoDSC.vi"("error in (no error)"=w1202, "Response"=w1201) -> ("error out"=w1190:errorcluster)  [unwired: 9 in]
        n550 = call "MercuryStateHistory.vi"("initialize?"=FALSE, "Current State in"=w1201) -> ("delimited string"=w1199:string)  [unwired: 8 in, 1 out]
        n551 = local write "Magnet Status 2"(w1199) -> ()
        n552 = call <userlib>:"FGV_PSP - Mercury Actions.vi"("error in"=w1190, "Function"=enum16{"write", "read"}."read") -> ("error out"=w1191:errorcluster, "Actions"=w1192:T52)  [unwired: 4 in]
        n553 = Bundle By Name(cluster=w1192, "Lambda"=w1195) -> (w1196:T52)
        n554 = call <userlib>:"FGV_PSP - Mercury Actions.vi"("error in"=w1191, "Function"=enum16{"write", "read"}."write", "Actions"=w1196) -> ("error out"=w1194:errorcluster)  [unwired: 3 in, 1 out]
        n555 = call <vilib>:"Add State(s) to Queue__JKI_lib_State_Machine.vi"("State(s) in (\"\")"=w1210) -> ("States Out"=w1211:string)  [unwired: 14 in]
      }
      frame "Mercury: Fast/Slow Fill" {
        n556 = local read "IPS Devices"() -> (w1229:string[])
        n557 = Unbundle By Name(w1215) -> ("Mercury IPS Ref"=w1231:T36)
        n558 = local read "Fast/Slow Fill"() -> (w1216:bool)
        n559 = Index Array(array=w1229, index=0) -> (element=w1224:string)
        n560 = call-poly <instrlib>:"Open.vi"("error in (no error)"=w1218, "Device Identifier"=w1224, "Mercury Reference In"=w1231) -> ("error out"=w1226:errorcluster, "Mercury Reference Out"=w1227:T36)  [unwired: 7 out]
        n561 = Select(t="OFF" ("Temperature setpoint"), s=w1216, f="ON" ("Temperature setpoint")) -> (s? t:f=w1228:string)
        n562 = call-poly <instrlib>:"Configuration (Set).vi"("ISOBUS address"=T34 -1, "error in"=w1226, "Delay"=w1228, "Mercury Reference In"=w1227) -> ("error out"=w1220:errorcluster, "Response"=w1219:T35)  [unwired: 4 in, 2 out]
        n563 = call "MercuryStateHistory.vi"("Current State in"=w1219) -> ("delimited string"=w1221:string)  [unwired: 9 in, 1 out]
        n564 = call "IPSReplytoDSC.vi"("error in (no error)"=w1220, "Response"=w1219) -> ("error out"=w1217:errorcluster)  [unwired: 9 in]
        n565 = local write "Magnet Status 2"(w1221) -> ()
        n566 = call <vilib>:"Add State(s) to Queue__JKI_lib_State_Machine.vi"("State(s) in (\"\")"=w1232) -> ("States Out"=w1233:string)  [unwired: 14 in]
      }
      frame "Mercury: Needle Valve" {
        n567 = Unbundle By Name(w1236) -> ("Mercury ITC Ref"=w1248:T36)
        n568 = Build Array("Close Needle Valve", "Open Needle Valve") -> (w1244:bool[])
        n569 = call-poly <instrlib>:"Open.vi"("error in (no error)"=w1234, "Device Identifier"="lambda:LPC", "Mercury Reference In"=w1248) -> ("error out"=w1243:errorcluster, "Mercury Reference Out"=w1242:T36)  [unwired: 7 out]
        n570 = Boolean Array To Number(Boolean array=w1244) -> (number=w1241:u32)
        n571 = case shown="1" w1241 {
          tunnel: w1243 -> [w1253 w1257 w1266]
          tunnel: w1242 -> [_ w1258 w1265]
          tunnel: [w1253 w1256 w1264] -> w1238
          tunnel: [T35 "" ("Response") w1255 w1263] -> w1237
          tunnel: [FALSE ("Close Needle Valve") FALSE ("Close Needle Valve") FALSE ("Close Needle Valve")] -> w1240
          frame 0, Default {
          }
          frame 1 {
            n572 = call-poly <instrlib>:"Configuration (Set).vi"("ISOBUS address"=T34 -1, "error in"=w1257, "Percentage Open"=0.0, "Mercury Reference In"=w1258) -> ("error out"=w1256:errorcluster, "Response"=w1255:T35)  [unwired: 4 in, 2 out]
          }
          frame 2 {
            n573 = call-poly <instrlib>:"Configuration (Set).vi"("ISOBUS address"=T34 -1, "error in"=w1266, "Percentage Open"="Percentage Open", "Mercury Reference In"=w1265) -> ("error out"=w1264:errorcluster, "Response"=w1263:T35)  [unwired: 4 in, 2 out]
          }
        }
        n574 = local write "Close Needle Valve"(w1240) -> ()
        n575 = local write "Open Needle Valve"(w1240) -> ()
        n576 = call "ITCReplytoDSC.vi"("error in (no error)"=w1238, "Response"=w1237) -> ("error out"=w1235:errorcluster)  [unwired: 9 in]
        n577 = call "MercuryStateHistory.vi"("Current State in"=w1237) -> ("delimited string"=w1239:string)  [unwired: 9 in, 1 out]
        n578 = local write "Magnet Status 2"(w1239) -> ()
        n579 = call <vilib>:"Add State(s) to Queue__JKI_lib_State_Machine.vi"("State(s) in (\"\")"=w1249) -> ("States Out"=w1250:string)  [unwired: 14 in]
      }
    }
  }
  n580 = disable-structure shown="Disabled" {
    frame Disabled {
      (unwired) FALSE
      n581 = call-poly <instrlib>:"Configuration (Read).vi"() -> ()  [unwired: 3 in, 9 out]
      n582 = disable-structure shown="Disabled" {
        frame Disabled {
          n583 = property on="Fast/Slow Fill" class="Bool (strict)" props=["Val(Sgnl)"]() -> ()  [unwired: 3 in, 2 out]
        }
        frame Enabled {
        }
      }
      n584 = local read "PS Heat"() -> ()  [unwired: 1 in]
      n585 = local read "Lambda"() -> ()  [unwired: 1 in]
      n586 = call-poly <instrlib>:"Signals (Read).vi"() -> ()  [unwired: 3 in, 9 out]
    }
    frame Enabled {
    }
  }
